vi "Text control 2 v4.8_pump-specific.vi"() -> ()   [LabVIEW 2016]
panel:
  in  "Tab Control":enum32{"Main", "Other parameters"}(tab)
  out "Line running":i32
  out "Total lines":i32
  out "Path":path=path "C:/users/rlp38/09Apr2009LTtesting/test2.txt"
  out "I vs Vg":cluster{"Y data in":dbl[], "X data in":dbl[]}[](graph)
  out "Is":dbl format="%.2e"
  out "Id":dbl format="%.2e"
  out "Ig":dbl format="%.2e"
  out "Id max vs time":cluster{"Y data in":dbl[], "X data in":dbl[]}[](graph)
  out "Id min vs time":cluster{"Y data in":dbl[], "X data in":dbl[]}[](graph)
  out "I vs Vd":cluster{"Y data in":dbl[], "X data in":dbl[]}[](graph)
  in  "Program":string="# Set time units to minutes.\n# Change filenames\n#-------------------------------------------------------\n# Port settings\n# Port 1: Nothing\n# Port 2: To sample\n# Port 3: Ultrapure water\n# Port 4: Nothing\n# Port 5: Nothing\n# Port 6: Nothing\n#-------------------------------------------------------\n# Execution time: 4 x 30 = 120 minutes = 2 hours\n# This script is designed to perform a cycling experiment between two liquids.\n# There are 4 pumping cycles, each one followed by 30 minutes of measurements.\n# All cycles pump ultrapure water (port 3).\n# Flow V = 20 pulses/second (400 ul/min)\n#-------------------------------------------------------\n# Cycle 1\npump /1ZR #initialize pump\npump /1Q #query pump\npump /1? #report absolute plunger position\ntransfer d 1 -1 -0.1 -1 -1 0\nwait-min 1 #wait 1 minute\npump /1N0R #set step resolution: 0.01 mm\npump /1Q #query pump\npump /1? #report absolute plunger position #the plunger should be at 0\nwait 1000 #wait 1 second\npump /1V300R #choose speed: 300 steps/s\npump /1Q #query pump\nwait 1000 #wait 1 second\npump /1O3R #go to port 3, counterclockwise rotation\npump /1Q #query pump\nwait 1000 #wait 1 second\npump /1A2400R #go to absolute position 2400\nwait 20000 #wait 20 seconds\npump /1V20R #set speed to 20 steps/s\npump /1Q #query pump\nwait 10000 # wait 10 seconds\npump /1? #report absolute plunger position #the plunger should have finished moving\npump /1O2R #switch to port 2, counterclockwise rotation\npump /1Q #query pump\nwait 200 #wait 200 milliseconds\npump /1A0R #go to absolute position 0 (= empty syringe)\npump /1Q #query pump\ntransfer d 1 -1 -0.1 -1 -1 0\nwait-min 1\npump /1Q #query pump\npump /1? #report absolute plunger position\ntransfer d 1 -1 -0.1 -1 -1 0\nwait-min 1\npump /1Q #query pump\npump /1? #report absolute plunger position\ntransfer d 1 -1 -0.1 -1 -1 0\nwait-min 1\npump /1Q #query pump\npump /1? #report absolute plunger position\ntransfer d 1 -1 -0.1 -1 -1 0\nwait-min 1\npump /1Q #query pump\npump /1? #report absolute plunger position\ntransfer d 1 -1 -0.1 -1 -1 0\nwait-min 1\npump /1Q #query pump\npump /1? #report absolute plunger position\ntransfer d 1 -1 -0.1 -1 -1 0\nwait-min 1\npump /1Q #query pump\npump /1? #report absolute plunger position\ntransfer d 1 -1 -0.1 -1 -1 0\nwait-min 1\npump /1Q #query pump\npump /1? #report absolute plunger position\ntransfer d 1 -1 -0.1 -1 -1 0\nwait-min 1\npump /1Q #query pump\npump /1? #report absolute plunger position\ntransfer d 1 -1 -0.1 -1 -1 0\nwait-min 1\npump /1Q #query pump\npump /1? #report absolute plunger position\ntransfer d 1 -1 -0.1 -1 -1 0\nwait-min 1\npump /1Q #query pump\npump /1? #report absolute plunger position\ntransfer d 1 -1 -0.1 -1 -1 0\nwait-min 1\npump /1Q #query pump\npump /1? #report absolute plunger position\ntransfer d 1 -1 -0.1 -1 -1 0\nwait-min 1\npump /1Q #query pump\npump /1? #report absolute plunger position\ntransfer d 1 -1 -0.1 -1 -1 0\nwait-min 1\npump /1Q #query pump\npump /1? #report absolute plunger position\ntransfer d 1 -1 -0.1 -1 -1 0\nwait-min 1\npump /1Q #query pump\npump /1? #report absolute plunger position\ntransfer d 1 -1 -0.1 -1 -1 0\nwait-min 1\npump /1Q #query pump\npump /1? #report absolute plunger position\ntransfer d 1 -1 -0.1 -1 -1 0\nwait-min 1\npump /1Q #query pump\npump /1? #report absolute plunger position\ntransfer d 1 -1 -0.1 -1 -1 0\nwait-min 1\npump /1Q #query pump\npump /1? #report absolute plunger position\ntransfer d 1 -1 -0.1 -1 -1 0\nwait-min 1\npump /1Q #query pump\npump /1? #report absolute plunger position\ntransfer d 1 -1 -0.1 -1 -1 0\nwait-min 1\npump /1Q #query pump\npump /1? #report absolute plunger position\ntransfer d 1 -1 -0.1 -1 -1 0\nwait-min 1\npump /1Q #query pump\npump /1? #report absolute plunger position\ntransfer d 1 -1 -0.1 -1 -1 0\nwait-min 1\npump /1Q #query pump\npump /1? #report absolute plunger position\ntransfer d 1 -1 -0.1 -1 -1 0\nwait-min 1\npump /1Q #query pump\npump /1? #report absolute plunger position\ntransfer d 1 -1 -0.1 -1 -1 0\nwait-min 1\npump /1Q #query pump\npump /1? #report absolute plunger position\ntransfer d 1 -1 -0.1 -1 -1 0\nwait-min 1\npump /1Q #query pump\npump /1? #report absolute plunger position\ntransfer d 1 -1 -0.1 -1 -1 0\nwait-min 1\n#-------------------------------------------------------\n# Cycle 2\npump /1ZR #initialize pump\npump /1Q #query pump\npump /1? #report absolute plunger position\ntransfer d 1 -1 -0.1 -1 -1 0\nwait-min 1 #wait 1 minute\npump /1N0R #set step resolution: 0.01 mm\npump /1Q #query pump\npump /1? #report absolute plunger position #the plunger should be at 0\nwait 1000 #wait 1 second\npump /1V300R #choose speed: 300 steps/s\npump /1Q #query pump\nwait 1000 #wait 1 second\npump /1O3R #go to port 3, counterclockwise rotation\npump /1Q #query pump\nwait 1000 #wait 1 second\npump /1A2400R #go to absolute position 2400\nwait 20000 #wait 20 seconds\npump /1V20R #set speed to 20 steps/s\npump /1Q #query pump\nwait 10000 # wait 10 seconds\npump /1? #report absolute plunger position #the plunger should have finished moving\npump /1O2R #switch to port 2, counterclockwise rotation\npump /1Q #query pump\nwait 200 #wait 200 milliseconds\npump /1A0R #go to absolute position 0 (= empty syringe)\npump /1Q #query pump\npump /1? #report absolute plunger position #the plunger should be moving to 0\ntransfer d 1 -1 -0.1 -1 -1 0\nwait-min 1\npump /1Q #query pump\npump /1? #report absolute plunger position\ntransfer d 1 -1 -0.1 -1 -1 0\nwait-min 1\npump /1Q #query pump\npump /1? #report absolute plunger position\ntransfer d 1 -1 -0.1 -1 -1 0\nwait-min 1\npump /1Q #query pump\npump /1? #report absolute plunger position\ntransfer d 1 -1 -0.1 -1 -1 0\nwait-min 1\npump /1Q #query pump\npump /1? #report absolute plunger position\ntransfer d 1 -1 -0.1 -1 -1 0\nwait-min 1\npump /1Q #query pump\npump /1? #report absolute plunger position\ntransfer d 1 -1 -0.1 -1 -1 0\nwait-min 1\npump /1Q #query pump\npump /1? #report absolute plunger position\ntransfer d 1 -1 -0.1 -1 -1 0\nwait-min 1\npump /1Q #query pump\npump /1? #report absolute plunger position\ntransfer d 1 -1 -0.1 -1 -1 0\nwait-min 1\npump /1Q #query pump\npump /1? #report absolute plunger position\ntransfer d 1 -1 -0.1 -1 -1 0\nwait-min 1\npump /1Q #query pump\npump /1? #report absolute plunger position\ntransfer d 1 -1 -0.1 -1 -1 0\nwait-min 1\npump /1Q #query pump\npump /1? #report absolute plunger position\ntransfer d 1 -1 -0.1 -1 -1 0\nwait-min 1\npump /1Q #query pump\npump /1? #report absolute plunger position\ntransfer d 1 -1 -0.1 -1 -1 0\nwait-min 1\npump /1Q #query pump\npump /1? #report absolute plunger position\ntransfer d 1 -1 -0.1 -1 -1 0\nwait-min 1\npump /1Q #query pump\npump /1? #report absolute plunger position\ntransfer d 1 -1 -0.1 -1 -1 0\nwait-min 1\npump /1Q #query pump\npump /1? #report absolute plunger position\ntransfer d 1 -1 -0.1 -1 -1 0\nwait-min 1\npump /1Q #query pump\npump /1? #report absolute plunger position\ntransfer d 1 -1 -0.1 -1 -1 0\nwait-min 1\npump /1Q #query pump\npump /1? #report absolute plunger position\ntransfer d 1 -1 -0.1 -1 -1 0\nwait-min 1\npump /1Q #query pump\npump /1? #report absolute plunger position\ntransfer d 1 -1 -0.1 -1 -1 0\nwait-min 1\npump /1Q #query pump\npump /1? #report absolute plunger position\ntransfer d 1 -1 -0.1 -1 -1 0\nwait-min 1\npump /1Q #query pump\npump /1? #report absolute plunger position\ntransfer d 1 -1 -0.1 -1 -1 0\nwait-min 1\npump /1Q #query pump\npump /1? #report absolute plunger position\ntransfer d 1 -1 -0.1 -1 -1 0\nwait-min 1\npump /1Q #query pump\npump /1? #report absolute plunger position\ntransfer d 1 -1 -0.1 -1 -1 0\nwait-min 1\npump /1Q #query pump\npump /1? #report absolute plunger position\ntransfer d 1 -1 -0.1 -1 -1 0\nwait-min 1\npump /1Q #query pump\npump /1? #report absolute plunger position\ntransfer d 1 -1 -0.1 -1 -1 0\nwait-min 1\npump /1Q #query pump\npump /1? #report absolute plunger position\ntransfer d 1 -1 -0.1 -1 -1 0\nwait-min 1\n#-------------------------------------------------------\n# Cycle 3\npump /1ZR #initialize pump\npump /1Q #query pump\npump /1? #report absolute plunger position\ntransfer d 1 -1 -0.1 -1 -1 0\nwait-min 1 #wait 1 minute\npump /1N0R #set step resolution: 0.01 mm\npump /1Q #query pump\npump /1? #report absolute plunger position #the plunger should be at 0\nwait 1000 #wait 1 second\npump /1V300R #choose speed: 300 steps/s\npump /1Q #query pump\nwait 1000 #wait 1 second\npump /1O3R #go to port 3, counterclockwise rotation\npump /1Q #query pump\nwait 1000 #wait 1 second\npump /1A2400R #go to absolute position 2400\nwait 20000 #wait 20 seconds\npump /1V20R #set speed to 20 steps/s\npump /1Q #query pump\nwait 10000 # wait 10 seconds\npump /1? #report absolute plunger position #the plunger should have finished moving\npump /1O2R #switch to port 2, counterclockwise rotation\npump /1Q #query pump\nwait 200 #wait 200 milliseconds\npump /1A0R #go to absolute position 0 (= empty syringe)\npump /1Q #query pump\npump /1? #report absolute plunger position #the plunger should be moving to 0\ntransfer d 1 -1 -0.1 -1 -1 0\nwait-min 1\npump /1Q #query pump\npump /1? #report absolute plunger position\ntransfer d 1 -1 -0.1 -1 -1 0\nwait-min 1\npump /1Q #query pump\npump /1? #report absolute plunger position\ntransfer d 1 -1 -0.1 -1 -1 0\nwait-min 1\npump /1Q #query pump\npump /1? #report absolute plunger position\ntransfer d 1 -1 -0.1 -1 -1 0\nwait-min 1\npump /1Q #query pump\npump /1? #report absolute plunger position\ntransfer d 1 -1 -0.1 -1 -1 0\nwait-min 1\npump /1Q #query pump\npump /1? #report absolute plunger position\ntransfer d 1 -1 -0.1 -1 -1 0\nwait-min 1\npump /1Q #query pump\npump /1? #report absolute plunger position\ntransfer d 1 -1 -0.1 -1 -1 0\nwait-min 1\npump /1Q #query pump\npump /1? #report absolute plunger position\ntransfer d 1 -1 -0.1 -1 -1 0\nwait-min 1\npump /1Q #query pump\npump /1? #report absolute plunger position\ntransfer d 1 -1 -0.1 -1 -1 0\nwait-min 1\npump /1Q #query pump\npump /1? #report absolute plunger position\ntransfer d 1 -1 -0.1 -1 -1 0\nwait-min 1\npump /1Q #query pump\npump /1? #report absolute plunger position\ntransfer d 1 -1 -0.1 -1 -1 0\nwait-min 1\npump /1Q #query pump\npump /1? #report absolute plunger position\ntransfer d 1 -1 -0.1 -1 -1 0\nwait-min 1\npump /1Q #query pump\npump /1? #report absolute plunger position\ntransfer d 1 -1 -0.1 -1 -1 0\nwait-min 1\npump /1Q #query pump\npump /1? #report absolute plunger position\ntransfer d 1 -1 -0.1 -1 -1 0\nwait-min 1\npump /1Q #query pump\npump /1? #report absolute plunger position\ntransfer d 1 -1 -0.1 -1 -1 0\nwait-min 1\npump /1Q #query pump\npump /1? #report absolute plunger position\ntransfer d 1 -1 -0.1 -1 -1 0\nwait-min 1\npump /1Q #query pump\npump /1? #report absolute plunger position\ntransfer d 1 -1 -0.1 -1 -1 0\nwait-min 1\npump /1Q #query pump\npump /1? #report absolute plunger position\ntransfer d 1 -1 -0.1 -1 -1 0\nwait-min 1\npump /1Q #query pump\npump /1? #report absolute plunger position\ntransfer d 1 -1 -0.1 -1 -1 0\nwait-min 1\npump /1Q #query pump\npump /1? #report absolute plunger position\ntransfer d 1 -1 -0.1 -1 -1 0\nwait-min 1\npump /1Q #query pump\npump /1? #report absolute plunger position\ntransfer d 1 -1 -0.1 -1 -1 0\nwait-min 1\npump /1Q #query pump\npump /1? #report absolute plunger position\ntransfer d 1 -1 -0.1 -1 -1 0\nwait-min 1\npump /1Q #query pump\npump /1? #report absolute plunger position\ntransfer d 1 -1 -0.1 -1 -1 0\nwait-min 1\npump /1Q #query pump\npump /1? #report absolute plunger position\ntransfer d 1 -1 -0.1 -1 -1 0\nwait-min 1\npump /1Q #query pump\npump /1? #report absolute plunger position\ntransfer d 1 -1 -0.1 -1 -1 0\nwait-min 1\n#-------------------------------------------------------\n# Cycle 4\npump /1ZR #initialize pump\npump /1Q #query pump\npump /1? #report absolute plunger position\ntransfer d 1 -1 -0.1 -1 -1 0\nwait-min 1 #wait 1 minute\npump /1N0R #set step resolution: 0.01 mm\npump /1Q #query pump\npump /1? #report absolute plunger position #the plunger should be at 0\nwait 1000 #wait 1 second\npump /1V300R #choose speed: 300 steps/s\npump /1Q #query pump\nwait 1000 #wait 1 second\npump /1O3R #go to port 3, counterclockwise rotation\npump /1Q #query pump\nwait 1000 #wait 1 second\npump /1A2400R #go to absolute position 2400\nwait 20000 #wait 20 seconds\npump /1V20R #set speed to 20 steps/s\npump /1Q #query pump\nwait 10000 # wait 10 seconds\npump /1? #report absolute plunger position #the plunger should have finished moving\npump /1O2R #switch to port 2, counterclockwise rotation\npump /1Q #query pump\nwait 200 #wait 200 milliseconds\npump /1A0R #go to absolute position 0 (= empty syringe)\npump /1Q #query pump\npump /1? #report absolute plunger position #the plunger should be moving to 0\ntransfer d 1 -1 -0.1 -1 -1 0\nwait-min 1\npump /1Q #query pump\npump /1? #report absolute plunger position\ntransfer d 1 -1 -0.1 -1 -1 0\nwait-min 1\npump /1Q #query pump\npump /1? #report absolute plunger position\ntransfer d 1 -1 -0.1 -1 -1 0\nwait-min 1\npump /1Q #query pump\npump /1? #report absolute plunger position\ntransfer d 1 -1 -0.1 -1 -1 0\nwait-min 1\npump /1Q #query pump\npump /1? #report absolute plunger position\ntransfer d 1 -1 -0.1 -1 -1 0\nwait-min 1\npump /1Q #query pump\npump /1? #report absolute plunger position\ntransfer d 1 -1 -0.1 -1 -1 0\nwait-min 1\npump /1Q #query pump\npump /1? #report absolute plunger position\ntransfer d 1 -1 -0.1 -1 -1 0\nwait-min 1\npump /1Q #query pump\npump /1? #report absolute plunger position\ntransfer d 1 -1 -0.1 -1 -1 0\nwait-min 1\npump /1Q #query pump\npump /1? #report absolute plunger position\ntransfer d 1 -1 -0.1 -1 -1 0\nwait-min 1\npump /1Q #query pump\npump /1? #report absolute plunger position\ntransfer d 1 -1 -0.1 -1 -1 0\nwait-min 1\npump /1Q #query pump\npump /1? #report absolute plunger position\ntransfer d 1 -1 -0.1 -1 -1 0\nwait-min 1\npump /1Q #query pump\npump /1? #report absolute plunger position\ntransfer d 1 -1 -0.1 -1 -1 0\nwait-min 1\npump /1Q #query pump\npump /1? #report absolute plunger position\ntransfer d 1 -1 -0.1 -1 -1 0\nwait-min 1\npump /1Q #query pump\npump /1? #report absolute plunger position\ntransfer d 1 -1 -0.1 -1 -1 0\nwait-min 1\npump /1Q #query pump\npump /1? #report absolute plunger position\ntransfer d 1 -1 -0.1 -1 -1 0\nwait-min 1\npump /1Q #query pump\npump /1? #report absolute plunger position\ntransfer d 1 -1 -0.1 -1 -1 0\nwait-min 1\npump /1Q #query pump\npump /1? #report absolute plunger position\ntransfer d 1 -1 -0.1 -1 -1 0\nwait-min 1\npump /1Q #query pump\npump /1? #report absolute plunger position\ntransfer d 1 -1 -0.1 -1 -1 0\nwait-min 1\npump /1Q #query pump\npump /1? #report absolute plunger position\ntransfer d 1 -1 -0.1 -1 -1 0\nwait-min 1\npump /1Q #query pump\npump /1? #report absolute plunger position\ntransfer d 1 -1 -0.1 -1 -1 0\nwait-min 1\npump /1Q #query pump\npump /1? #report absolute plunger position\ntransfer d 1 -1 -0.1 -1 -1 0\nwait-min 1\npump /1Q #query pump\npump /1? #report absolute plunger position\ntransfer d 1 -1 -0.1 -1 -1 0\nwait-min 1\npump /1Q #query pump\npump /1? #report absolute plunger position\ntransfer d 1 -1 -0.1 -1 -1 0\nwait-min 1\npump /1Q #query pump\npump /1? #report absolute plunger position\ntransfer d 1 -1 -0.1 -1 -1 0\nwait-min 1\npump /1Q #query pump\npump /1? #report absolute plunger position\ntransfer d 1 -1 -0.1 -1 -1 0\nwait-min 1\n#-------------------------------------------------------"
  out "Command running:":string="#output s 0 0 0 -0.008 0.008 0.002"
  out "Serial port data":string
  out "Elapsed Time":dbl caption="Elapsed Time (s)"
  in  "Units":u16(ring)=1 items=["Seconds", "Minutes", "Hours"]
  in  "Time Offset":dbl caption="Set Start Time (s)"
  in  "Reset":bool
  in  "Auto Reset":bool
  in  "integration time":u32(slide) max=2 step=1 scale=0.0..2.0
  in  "Interrupt run":bool
  out "Absolute plunger position vs time":cluster{"Y data in":dbl[], "X data in":dbl[]}[](graph)
  out "Valve position vs time":cluster{"Y data in":dbl[], "X data in":dbl[]}[](graph)
  in  "Halt pump":bool
  in  "Hard stop pump":bool
  in  "Gate Range\nmode":u16(ring) items=["Auto", "Limited", "Fixed"]
  in  "Gate Range":u8(slide)=6 max=11 scale=0.0..11.0
  in  "Source/Drain\nRange mode":u16(ring) items=["Auto", "Limited", "Fixed"]
  in  "Source/Drain Range":u8(slide)=6 max=11 scale=0.0..11.0
  in  "Panel Controls":T1={"Emergency Stop"=refnum, "TransGraph Max"=1e-05, "Text/Graph (text=false)"=TRUE} {"TransGraph Max" format="%.2e"}
  in  "Panel Controls 2":T2={"Emergency Stop"=refnum, "TransGraph Max"=1e-05, "Text/Graph (text=false)"=TRUE, "TransGraph Min"=1e-11} {"TransGraph Min" format="%.2e"; "TransGraph Max" format="%.2e"}
  in  "SMU4":cluster{"on/off":bool, "Voltage":dbl} {"Voltage" min=-100.0 max=100.0 format="%.2f"}
  in  "Full Reset":bool
  in  "Standby":T3
  out "error out":errorcluster
  in  "Delay before read (ms)":u32=1000
  in  "byte count":u32=64
  in  "Serial End Mode for Reads":u16(ring)=2 items=["None", "LastBit", "TermChar"]
  in  "Timeout (ms)":u32=10000
  in  "Enable Termination\nChar (T)":bool=TRUE
  in  "Termination char\n(0xA = '\\n' = LF)\n(0xD = '\\r' = CR)":u8=13 format="%.0x"
  in  "flow control":u16(ring) items=["None"=0, "XON/XOFF"=1, "RTS/CTS"=2, "DTR/DSR"=4]
  in  "stop bits":u16(ring)=10 items=["1.0"=10, "1.5"=15, "2.0"=20]
  in  "parity":u16(ring) items=["None", "Odd", "Even", "Mark", "Space"]
  in  "data bits":u16=8 min=5 max=8 step=1
  in  "VISA resource name":refnum<visa-resource-name>="COM6"
  in  "baud rate":u32=9600
  in  "Drain: Compliance":dbl=0.001 format="%.8f"
  in  "Gate: Compliance":dbl=0.001 format="%.8f"
  in  "hold time /s":dbl format="%.2f"
  in  "delay time /s":dbl format="%.2f"
  in  "Integration time (short)":dbl=0.0019 min=8e-05 max=0.0019 step=8e-05 format="%^.0e"
  in  "Integration time (long)":dbl=0.32 min=0.04 max=2.0 step=0.02 format="%.2f"
  in  "Step delay /s":dbl format="%.2f"
  in  "Prefix (transfer)":string="_step_1_ultrapure_H2O_"
  in  "Suffix (transfer)":string="_T.txt"
  in  "Prefix (Idmax-Idmin)":string="_step_1_ultrapure_H2O_Idmax_Idmin_vs_time_Vg=-1.0V_Vd=-1.0V"
  in  "Suffix (Idmax-Idmin)":string=".txt"
  in  "Prefix (output)":string="_step_1_ultrapure_H2O_"
  in  "Suffix (output)":string="_O.txt"
  in  "Prefix (script)":string="_step_1_ultrapure_H2O_script"
  in  "Prefix (serial port output)":string="_step_1_ultrapure_H2O_serial port output"
  in  "Prefix (plunger)":string="_step_1_ultrapure_H2O_plunger_vs_time"
  in  "Suffix (plunger)":string=".txt"
  in  "Gate":T4={"Gate Start"=0.0, "Gate Stop"=2.0, "Gate Step (linear only)"=1.0, "Gate Compliance"=0.0001, "Gate PComp"=0.0, "Range mode"=0, "Range"=6} {"Range" max=11 scale=0.0..11.0; "Range mode" items=["Auto", "Limited", "Fixed"]; "Gate PComp" format="%^.2e"; "Gate Compliance" format="%^.2e"; "Gate Step (linear only)" format="%^.4e"; "Gate Stop" format="%^.4e"; "Gate Start" format="%^.4e"}
  in  "Drain 2":T5={"Drain Start"=0.0, "Drain Stop"=2.0, "Drain Compliance"=0.0001, "Drain Step"=1.0, "Drain PComp"=0.0, "Range mode"=0, "Range"=6} {"Range" max=11 scale=0.0..11.0; "Range mode" items=["Auto", "Limited", "Fixed"]; "Drain PComp" format="%^.2e"; "Drain Step" format="%^.4e"; "Drain Compliance" format="%^.2e"; "Drain Stop" format="%^.4e"; "Drain Start" format="%^.4e"}
  in  "Timings 2":T6={"integration time"=0, "Short/Long integration time"=0.00064, "hold time (sec)"=0.0, "delay time (sec)"=0.0, "Step Time (0 disables)"=0.0, "sweep method"=0, "Pulse period"=0.005, "Base voltage"=0.0, "Pulse width"=0.0005} {"Pulse width" min=0.0005 max=0.1 step=0.0001 format="%.4f"; "Base voltage" format="%^.4e"; "Pulse period" min=0.005 max=1.0 step=0.0001 format="%.4f"; "sweep method" items=["Continuous", "Pulsed"]; "Step Time (0 disables)" format="%.2f"; "delay time (sec)" format="%.4f"; "hold time (sec)" format="%.4f"; "Short/Long integration time" format="%^.0e"; "integration time" scale=0.0..2.0}
  # "Syntax:\nitime [s|m|l]\ngaterangemode [a|l|f]\ndrainrangemode [a|l|f]\npulsed [on|off] PulsePeriod(sec) PulseBaseVoltage PulseONWidth(sec)\nstandby [on l off]\nwait NumMilliseconds\nwait-min NumMinutes\n# texthere = comment\ntransfer [s|d] VgStart VgStop VgStep VdStart VdStop VdStep\noutput [s|d] VgStart VgStop VgStep VdStart VdStop VdStep\nsample Vg Vd NumSamples Time(s) SampleInterval(s)\nsamplei Idg NumSamples Time(s) SampleInterval(s) VDGcompliance\n100 samples is approximately 13 seconds with medium integration\n# if in doubt use SampleInterval(s) = 0.004\nstressV VG VD IGcompliance IDcompliance Duration(sec)\nstressI IDG VDGcompliance Duration(sec)\nvsu2pulse Bias Duration(s)\npulsedstressV [s|d] VEstop VgON VgOFF Period(s) PulseONwidth(s) Vd\nsample-fpp Vg Vd NumSamples Time\nresample-fpp Vg Vd\ntransfer-fpp [s|d] VgStart VgStop VgStep VdStart VdStop VdStep\noutput-fpp [s|d] VgStart VgStop VgStep VdStart VdStop VdStep\nserial SerialPortCommand\npump SerialPortCommand for the OEM pump\n\nSPM OEM Pump Syntax (<x>: pump number, use 1 if only one pump):\nif the command syntax contains [R], then append the letter R to the command\n/<x>Q: query (a query command should follow each command)\n/<x>Z[R] or /<x>Y[R]: initialize pump\n/<x>N<n>[R] (<n>=0,1): <0> (<1>) microstep 0.01 mm (0.00125 mm) resolution\n/<x>I<n> (<n>=0-6): turn to port number n (clockwise)\n/<x>O<n> (<n>=0-6): turn to port number n (counterclockwise)\n/<x>X: Re-execute last command string\n/<x>G<n>[R] (<n>=0-60000): repeat command sequence (default: 0, 0=loop forever)\n/<x>g: Mark the start of a repeat sequence (max = 10)\n/<x>M<n>[R] (<n>=0-86400000): delay command execution by n milliseconds\n/<x>H: Halt; Pause the sequence after finishing the current move\n/<x>T: Hardstop; Interrupt the current move and suppress it from the sequence\n/<x>A<n>[R] (<n>=0-3000 with N=0, 0-24000 with N=1): absolute position\n/<x>P<n>[R] (<n>=0-3000 with N=0, 0-24000 with N=1): relative pickup\n/<x>D<n>[R] (<n>=0-3000 with N=0, 0-24000 with N=1): relative dispense\n/<x>V<n>[R] (<n>=5-1600 default: 150): set peak speed (pulses/sec)\n/<x>S<n>[R] (<n>=10-40 default: 22): set speed (NOT in pulses/sec, look in manual)\nNOTE: When controlled with absolute position, one does not need to pay special attention to the syringe that is mounted on the pump.\nWithdraw from lower stage (ports 3, 5), dispense from higher stage (ports 2, 4, 6).\nConnect Port 1 to waste."
  # "Time"
  # "1\n2\n3\n4\n5\n6\n7\n8\n9\n10\n11\n12\n13\n14\n15\n16\n17\n18\n19\n20"
  # "Serial port settings"
  # "Filename settings"
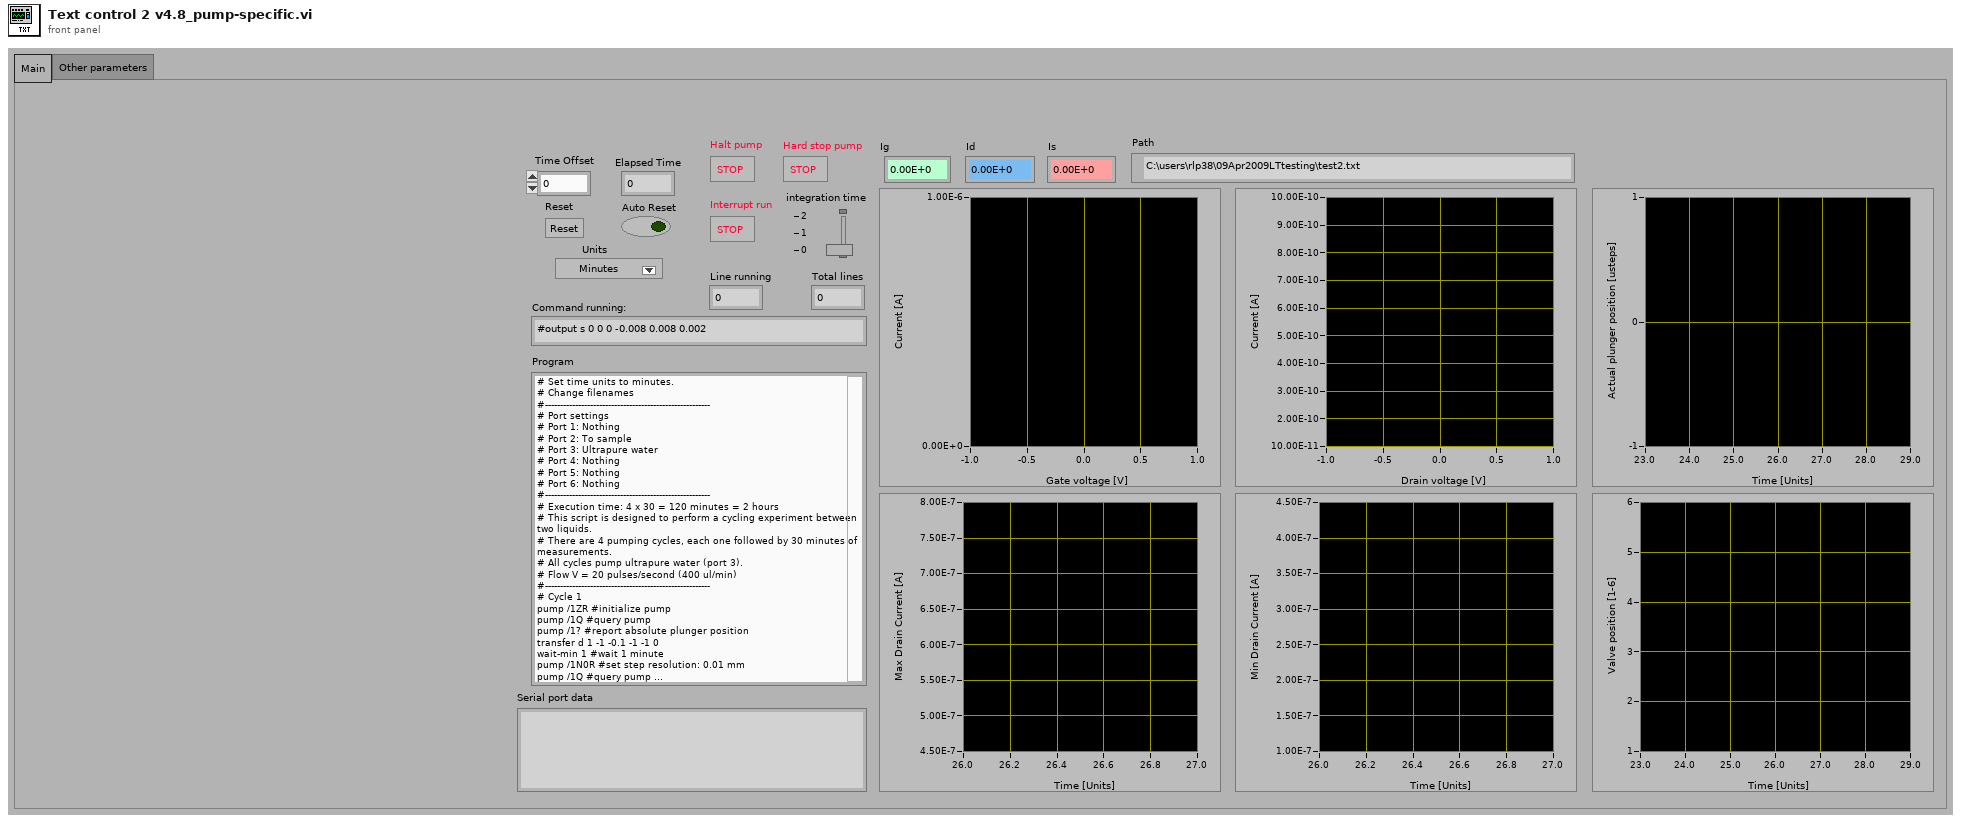
[diagram p1: front panel]
types:
  T1 = cluster{"Emergency Stop":refnum<vi>, "TransGraph Max":dbl, "Text/Graph (text=false)":bool}
  T2 = cluster{"Emergency Stop":refnum<vi>, "TransGraph Max":dbl, "Text/Graph (text=false)":bool, "TransGraph Min":dbl}
  T3 = cluster{"Gate Standby":bool, "Drain Standby":bool}
  T4 = cluster{"Gate Start":dbl, "Gate Stop":dbl, "Gate Step (linear only)":dbl, "Gate Compliance":dbl, "Gate PComp":dbl, "Range mode":u16, "Range":u8}
  T5 = cluster{"Drain Start":dbl, "Drain Stop":dbl, "Drain Compliance":dbl, "Drain Step":dbl, "Drain PComp":dbl, "Range mode":u16, "Range":u8}
  T6 = cluster{"integration time":u32, "Short/Long integration time":dbl, "hold time (sec)":dbl, "delay time (sec)":dbl, "Step Time (0 disables)":dbl, "sweep method":u16, "Pulse period":dbl, "Base voltage":dbl, "Pulse width":dbl}
  T7 = enum16{"open", "replace", "create", "open or create", "replace or create", "replace or create with confirmation"}
  T8 = cluster{"V2 Start":dbl, "V2 Step":dbl, "Number of points":i32}
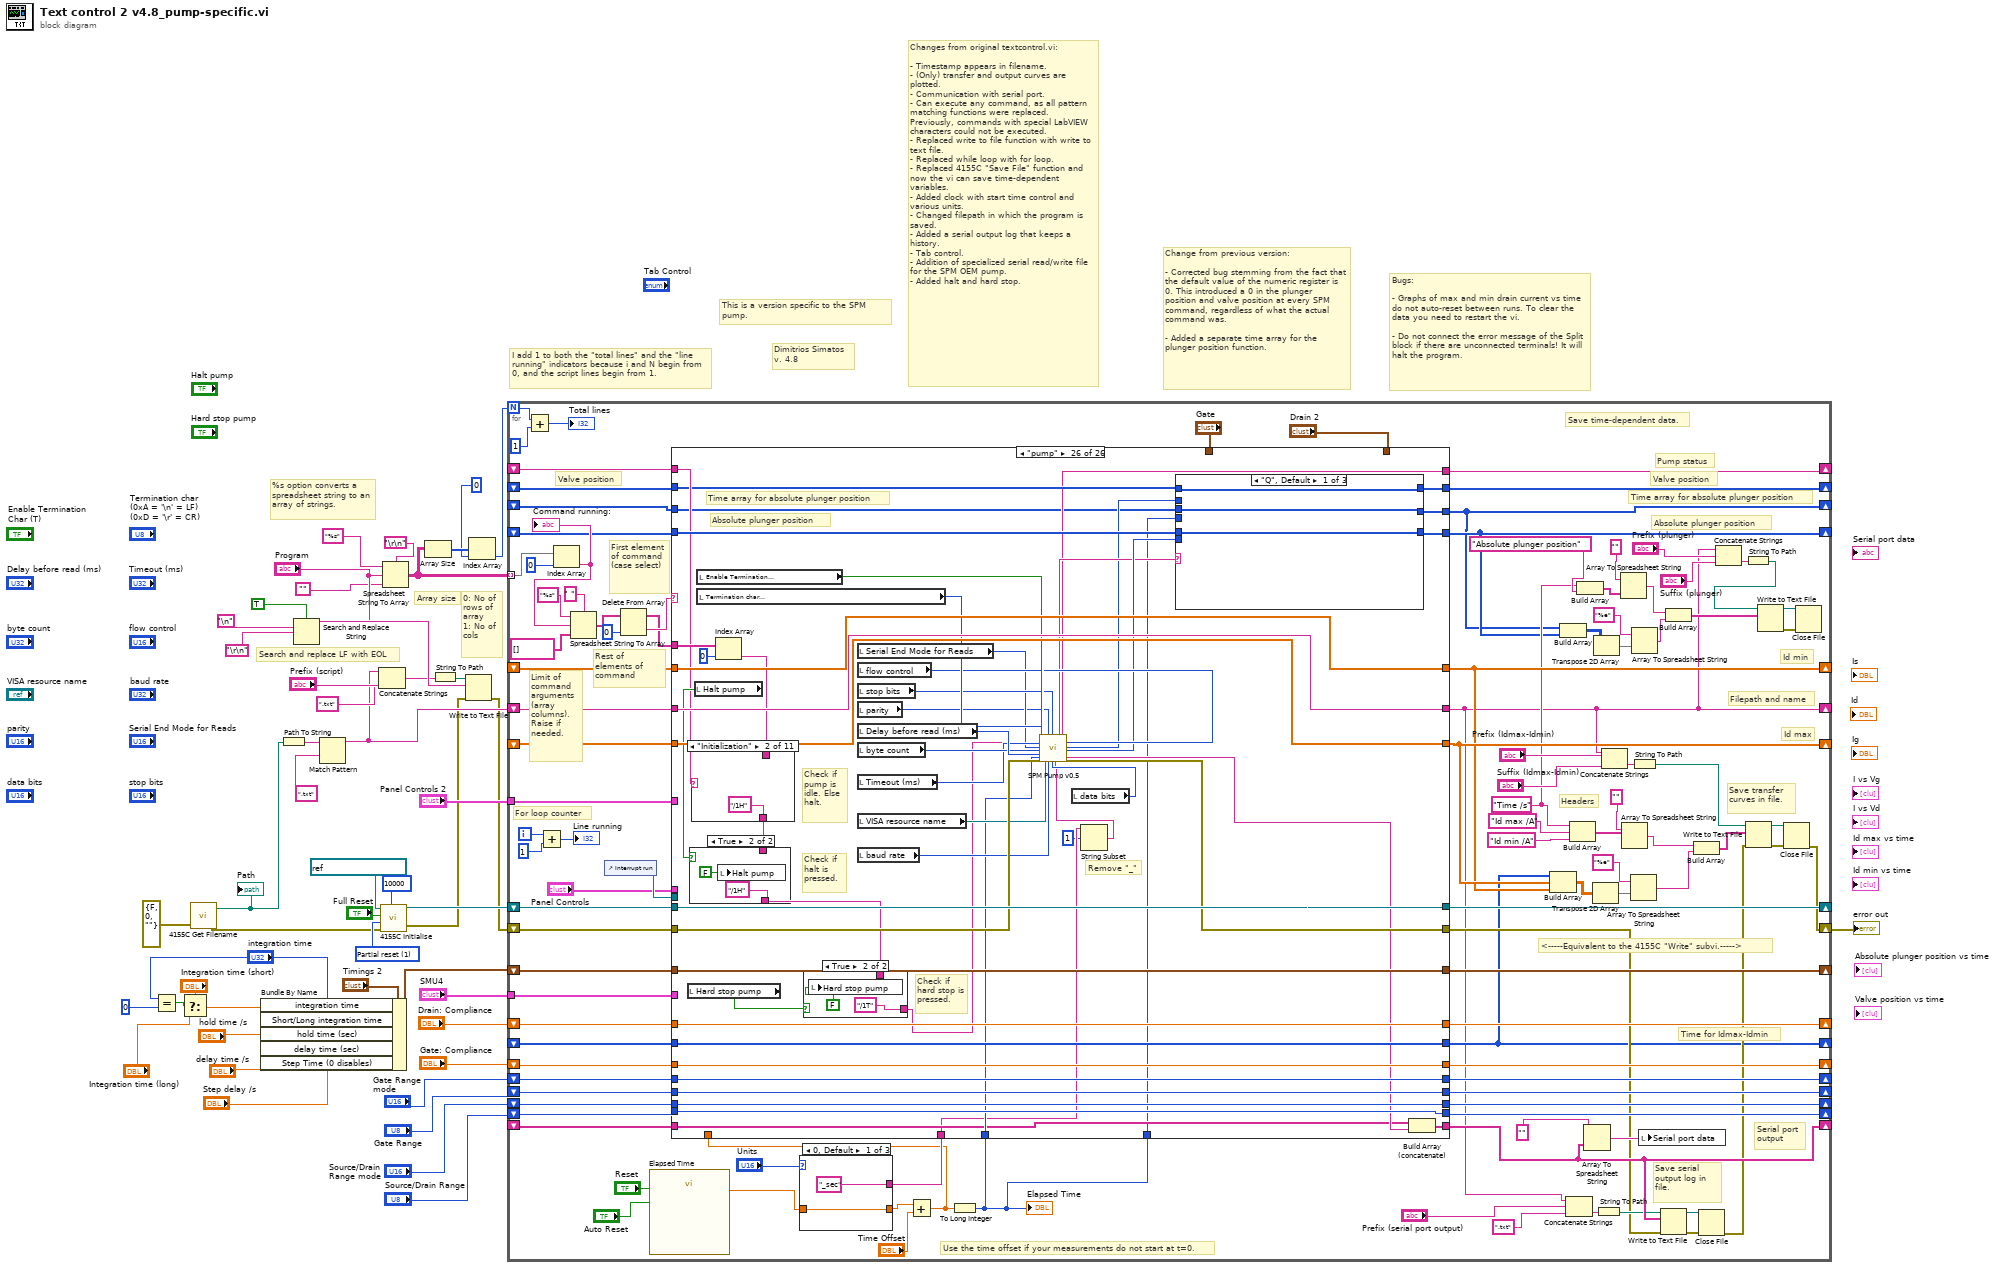
[diagram p0: block diagram]
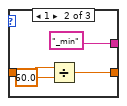
[diagram p2: hidden frame]
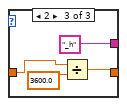
[diagram p3: hidden frame]
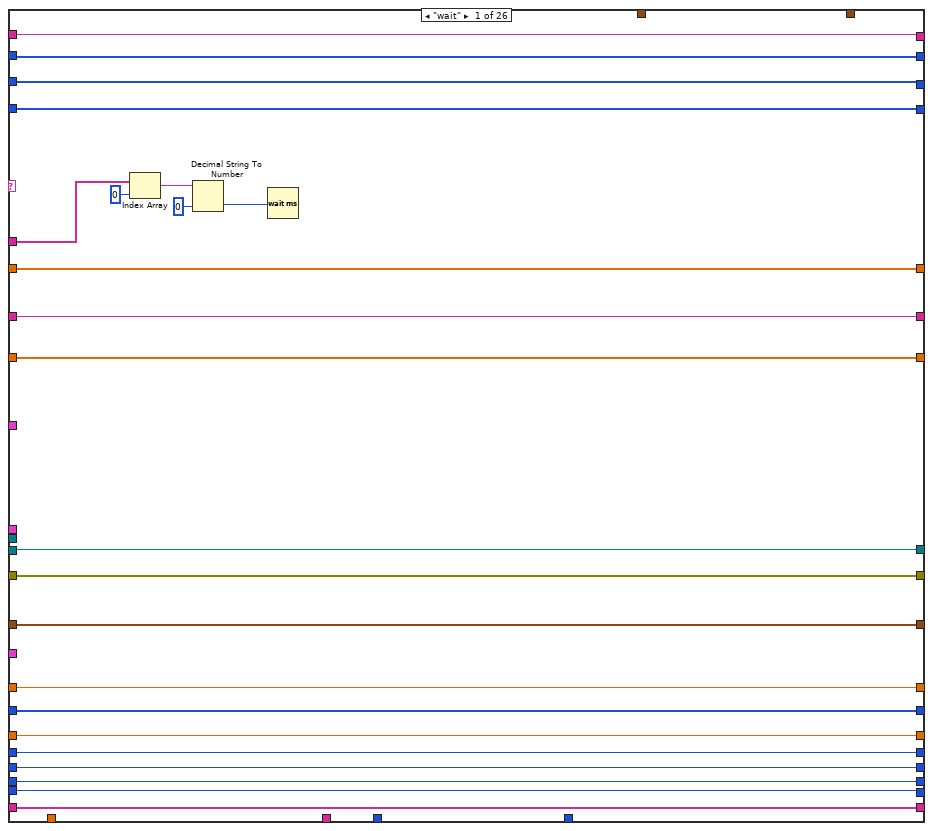
[diagram p4: hidden frame]
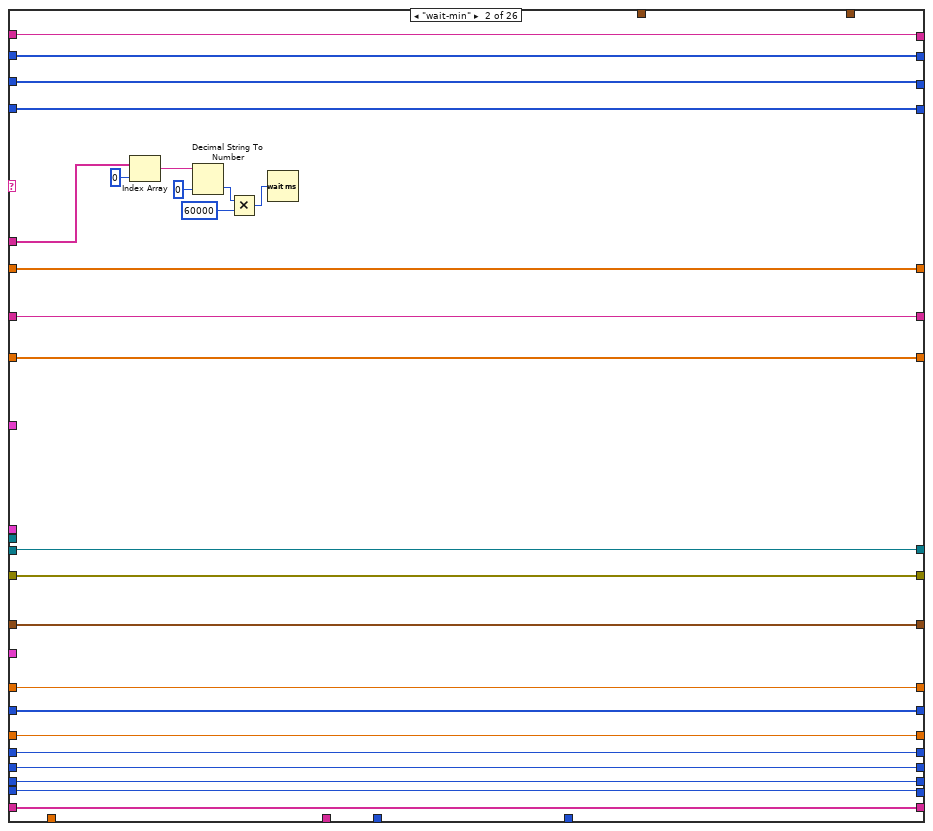
[diagram p5: hidden frame]
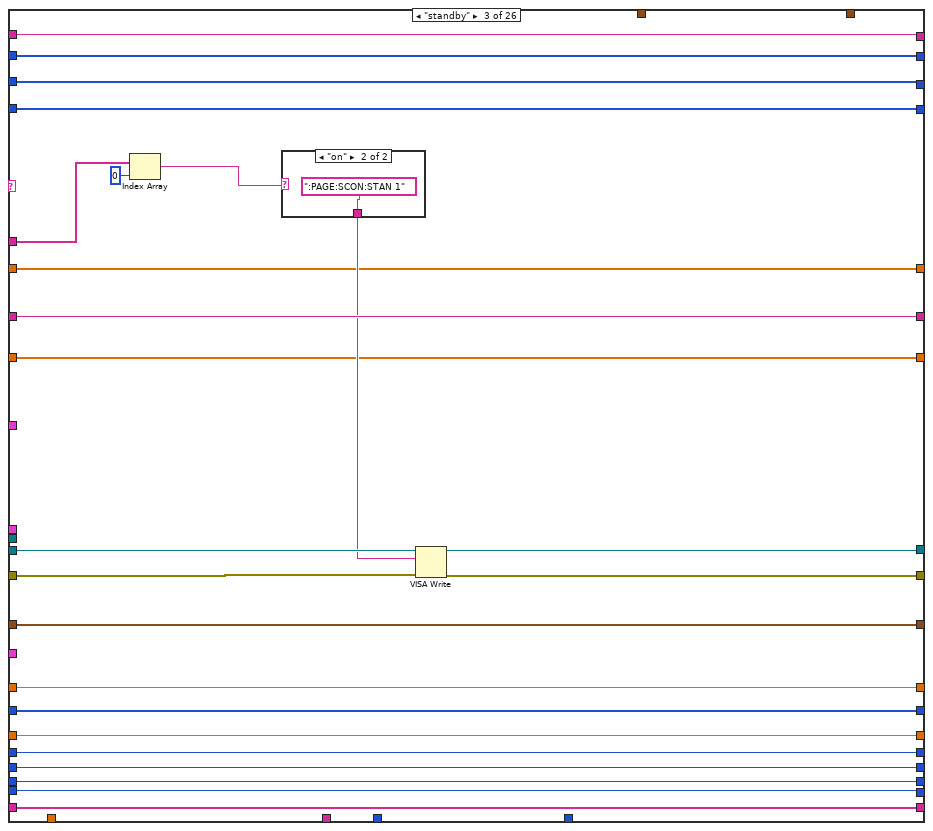
[diagram p6: hidden frame]
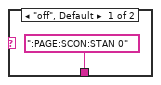
[diagram p7: hidden frame]
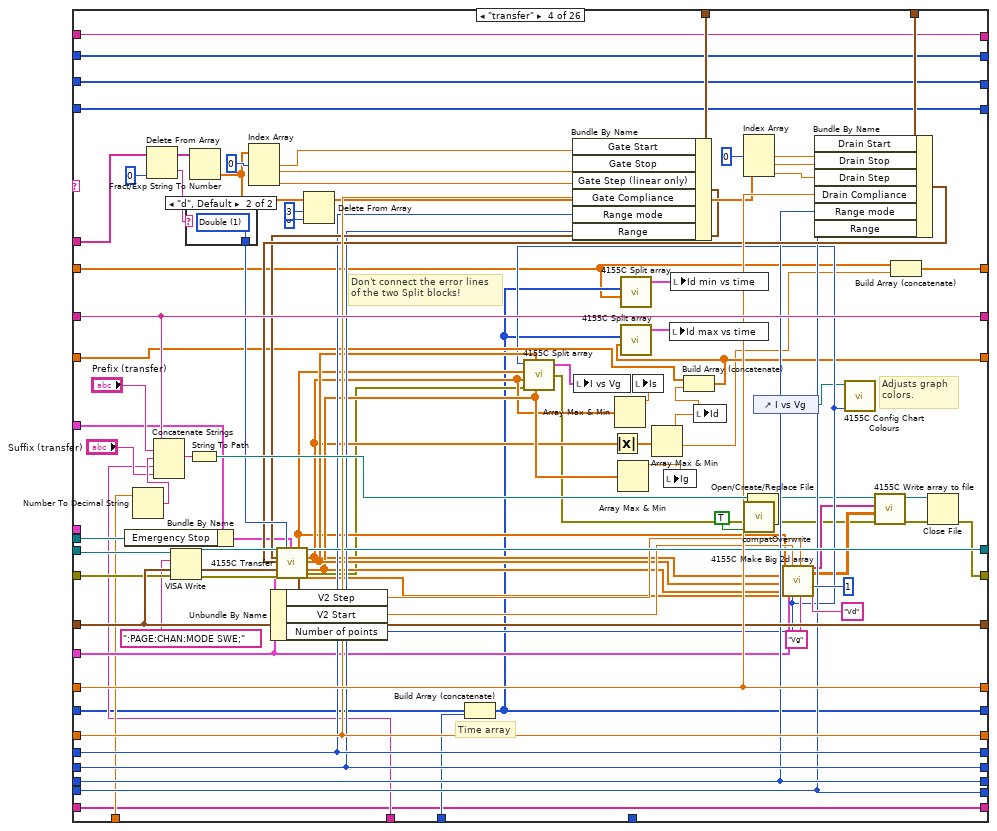
[diagram p8: hidden frame]
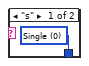
[diagram p9: hidden frame]
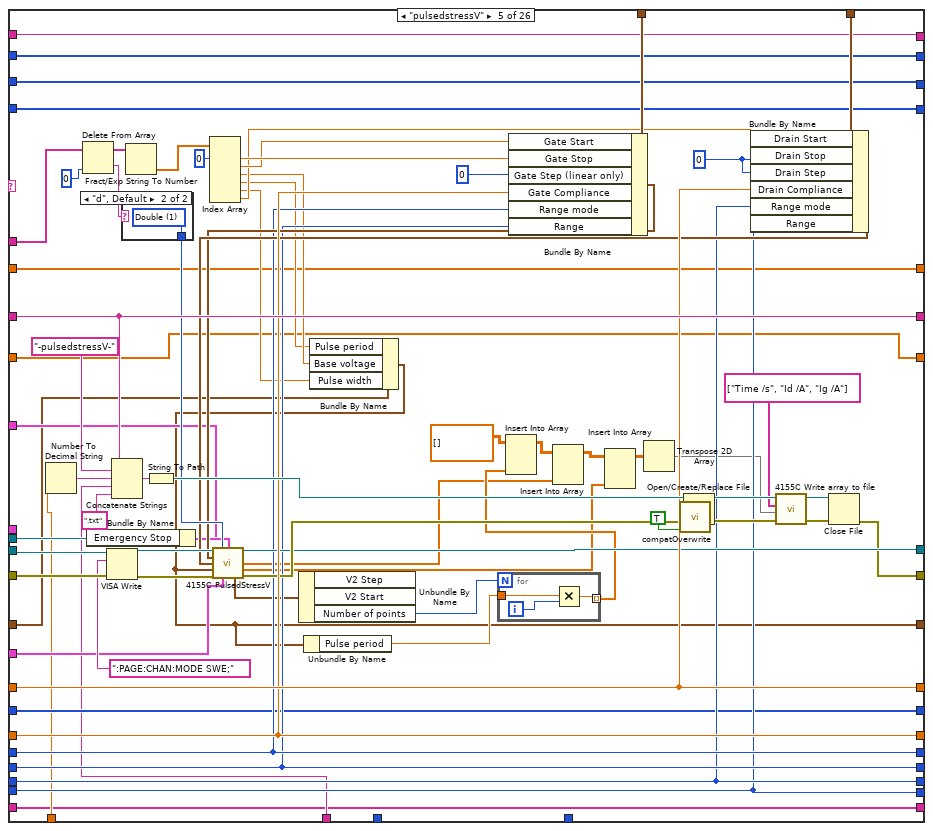
[diagram p10: hidden frame]
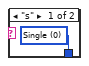
[diagram p11: hidden frame]
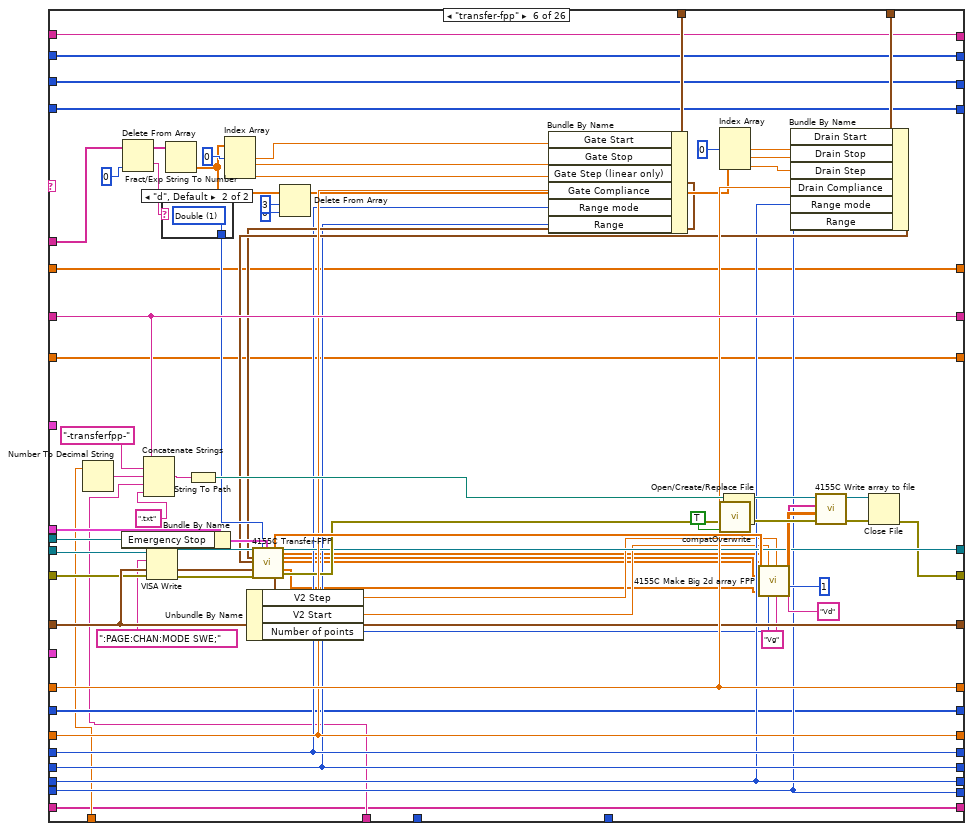
[diagram p12: hidden frame]
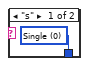
[diagram p13: hidden frame]
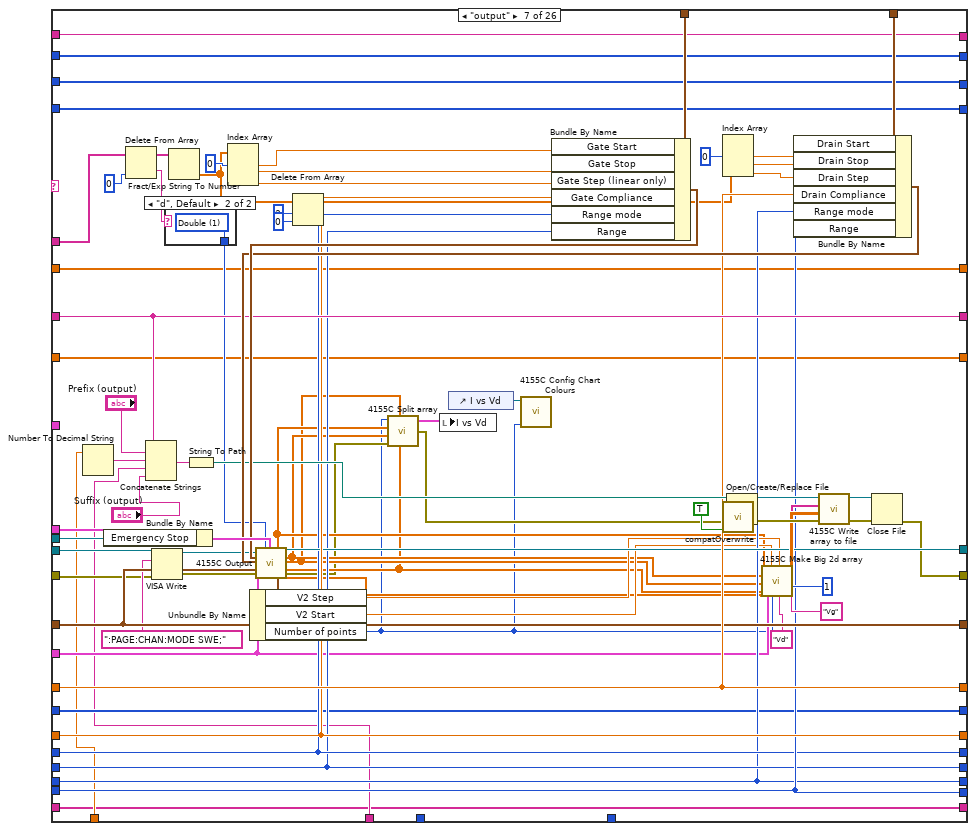
[diagram p14: hidden frame]
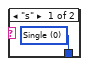
[diagram p15: hidden frame]
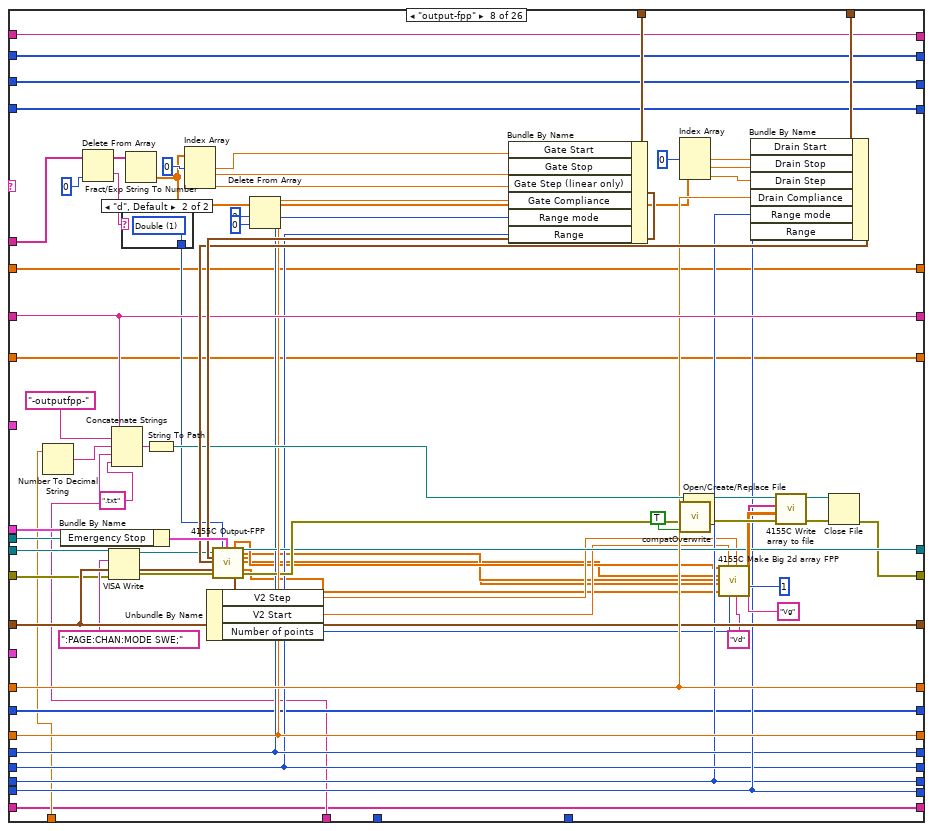
[diagram p16: hidden frame]
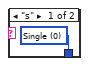
[diagram p17: hidden frame]
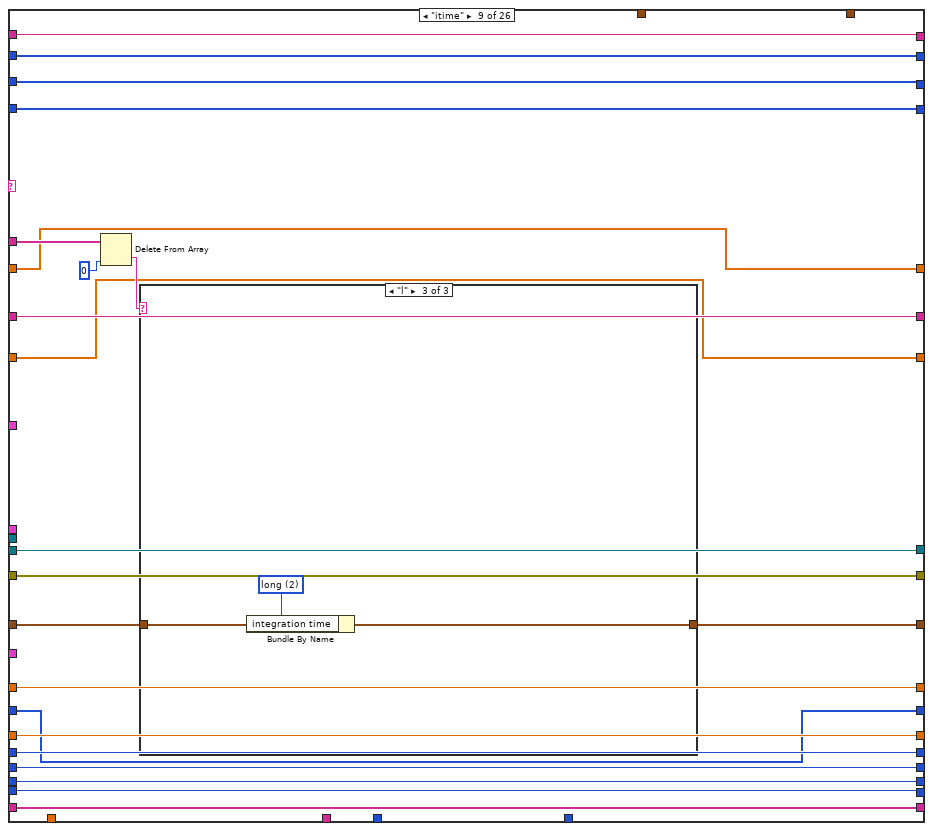
[diagram p18: hidden frame]
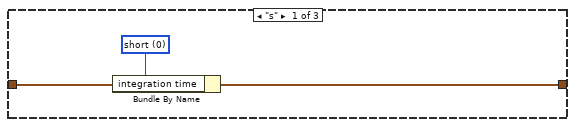
[diagram p19: hidden frame]
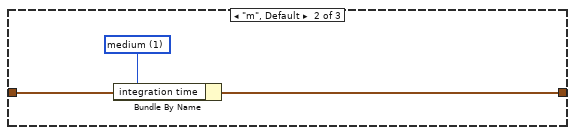
[diagram p20: hidden frame]
diagram:
  w40 = u16 1 items=["Reset All", "Partial reset"] ("Type of reset")
  # "Change from previous version:\n\n- Corrected bug stemming from the fact that the default value of the numeric register is 0. This introduced a 0 in the plunger position and valve position at every SPM command, regardless of what the actual command was.\n\n- Added a separate time array for the plunger position function."
  # "This is a version specific to the SPM pump."
  # "I add 1 to both the \"total lines\" and the \"line running\" indicators because i and N begin from 0, and the script lines begin from 1."
  # "Bugs:\n\n- Graphs of max and min drain current vs time do not auto-reset between runs. To clear the data you need to restart the vi.\n\n- Do not connect the error message of the Split block if there are unconnected terminals! It will halt the program."
  # "Array size"
  # "%s option converts a spreadsheet string to an array of strings."
  # "0: No of rows of array\n1: No of cols"
  # "Dimitrios Simatos\nv. 4.8"
  # "Changes from original textcontrol.vi:\n\n- Timestamp appears in filename.\n- (Only) transfer and output curves are plotted.\n- Communication with serial port.\n- Can execute any command, as all pattern matching functions were replaced. Previously, commands with special LabVIEW characters could not be executed.\n- Replaced write to file function with write to text file.\n- Replaced while loop with for loop.\n- Replaced 4155C \"Save File\" function and now the vi can save time-dependent variables.\n- Added clock with start time control and various units.\n- Changed filepath in which the program is saved.\n- Added a serial output log that keeps a history.\n- Tab control.\n- Addition of specialized serial read/write file for the SPM OEM pump.\n- Added halt and hard stop."
  # "Search and replace LF with EOL"
  n1 = Equal?(x="integration time", y=u32 0) -> (x = y?=w44:bool)
  n2 = Select(t="Integration time (short)", s=w44, f="Integration time (long)") -> (s? t:f=w48:dbl)
  n3 = call "4155C Get Filename.vi"("error in (no error)"=errorcluster {"status"=FALSE, "code"=0, "source"=""}) -> ("error out"=w35:errorcluster, "path"=w10:path)  [unwired: 2 in, 1 out]
  "Path" <- w10
  n4 = Bundle By Name(cluster="Timings 2", "integration time"="integration time", "Short/Long integration time"=w48, "hold time (sec)"="hold time /s", "delay time (sec)"="delay time /s", "Step Time (0 disables)"="Step delay /s") -> (w33:T6)
  n5 = Path To String(path=w10) -> (string=w11:string)
  n6 = Search and Replace String(replace all?=TRUE ("replace all? (F)"), input string="Program", search string="\n", replace string="\r\n") -> (result string=w23:string)  [unwired: 4 in, 3 out]
  n7 = Match Pattern(string=w11, regular expression=".txt") -> (before substring=w5:string)  [unwired: 1 in, 3 out]
  n8 = Concatenate Strings(w5, "Prefix (script)", ".txt" ("regular expression")) -> (w4:string)
  n9 = call "4155C Initialise.vi"("VISA resource name in"=refnum<visa-resource-name> "GPIB0::14::INSTR", "Reset"="Full Reset", "Type of reset"=w40, "error in (no error)"=w35, "VISA Timeout Value"=u32 10000) -> ("VISA Resource Name out"=w34:refnum<visa-resource-name>, "error out"=w2:errorcluster)
  n10 = Spreadsheet String To Array(delimiter (Tab)="\r\n", format string="%s", spreadsheet string="Program", array type (2D Dbl)="") -> (array=w14:string[][])
  n11 = Array Size(array=w14) -> (size(s)=w18:i32[])
  n12 = String To Path(string=w4) -> (path=w3:path)
  n13 = Write to Text File(file (use dialog)=w3, text=w23, error in=w2) -> (error out=w1:errorcluster)  [unwired: 1 in, 2 out]
  n14 = Index Array(array=w18, index=0) -> (element=w16:i32)
  n15 = for {
    N: w16 -> [w94]
    tunnel: "SMU4" -> [w136]
    shift-left: "Source/Drain Range" -> [w141]
    shift-right: [w137] -> _
    shift-left: "Source/Drain\nRange mode" -> [w142]
    shift-right: [w138] -> _
    shift-left: "Gate Range" -> [w143]
    shift-right: [w139] -> _
    shift-left: "Gate Range\nmode" -> [w144]
    shift-right: [w140] -> _
    shift-left: "Gate: Compliance" -> [w153]
    shift-right: [w149] -> _
    shift-left: "Drain: Compliance" -> [w154]
    shift-right: [w150] -> _
    shift-left: w33 -> [w155]
    shift-right: [w151] -> _
    shift-left: w1 -> [w156]
    shift-right: [w102] -> w9
    shift-left: w34 -> [w157]
    shift-right: [w152] -> _
    shift-left: w5 -> [w158]
    shift-right: [w53] -> _
    tunnel: "Panel Controls 2" -> [w135]
    shift-right: [w106] -> _
    shift-left: _ -> [w134]
    shift-right: [w55] -> _
    shift-left: _ -> [w130]
    tunnel: w14 -> [w129] mode=indexing
    shift-right: [w100] -> _
    shift-left: _ -> [w101]
    shift-right: [w83] -> _
    shift-left: _ -> [w86]
    shift-right: [w56] -> _
    shift-left: _ -> [w76]
    shift-right: [w75] -> _
    shift-left: _ -> [w74]
    shift-right: [w73] -> _
    shift-left: _ -> [w72]
    shift-right: [w50] -> _
    shift-left: _ -> [w51]
    i -> [w89]
    w57 = "Time /s" ("element")
    # "Time array for absolute plunger position"
    # "Valve position"
    # "Valve position"
    # "Pump status"
    # "Absolute plunger position"
    # "Serial port output"
    # "Save serial output log in file."
    # "For loop counter"
    # "<-----Equivalent to the 4155C \"Write\" subvi.----->"
    # "Headers"
    # "Save transfer curves in file."
    # "Filepath and name"
    # "Save time-dependent data."
    # "Use the time offset if your measurements do not start at t=0."
    # "Time for Idmax-Idmin"
    # "Rest of elements of command"
    # "Id min"
    # "Id max"
    # "Limit of command arguments (array columns). Raise if needed."
    # "First element of command\n(case select)"
    n16 = Add(x=w94, y=1) -> (x+y=→"Total lines":i32)
    n17 = Add(x=w89, y=1) -> (x+y=→"Line running":i32)
    n18 = Index Array(array=w129, index=0 ("line index")) -> (element=w124:string)
    "Command running:" <- w124
    n19 = Spreadsheet String To Array(delimiter (Tab)=" ", format string="%s", spreadsheet string=w124, array type (2D Dbl)=string[] []) -> (array=w121:string[])
    n20 = control-ref of="Interrupt run"() -> (w148:refnum<vi>)
    n21 = Delete From Array(array=w121, index=0) -> (deleted portion=w122:string, array with subset deleted=w120:string[])  [unwired: 1 in]
    n22 = call "Elapsed Time"("Reset"="Reset", "Auto Reset"="Auto Reset") -> ("Elapsed Time (s)"=w131:dbl)  [unwired: 10 in, 7 out]
    n23 = case shown="0, Default" "Units" {
      tunnel: ["_sec" "_min" "_h"] -> w132
      tunnel: [w159 w163 w166] -> w96
      tunnel: w131 -> [w159 w162 w167]
      frame 0, Default {
      }
      frame 1 {
        n24 = Divide(x=w162, y=60.0) -> (x/y=w163:dbl)
      }
      frame 2 {
        n25 = Divide(x=w167, y=3600.0) -> (x/y=w166:dbl)
      }
    }
    n26 = Add(x=w96, y="Time Offset") -> (x+y=w95:dbl)
    n27 = To Long Integer(number=w95) -> (32bit integer=w52:i32)
    "Elapsed Time" <- w52
    n28 = case shown="\"pump\"" w122 {
      tunnel: w120 -> [w191 w216 w240 w321 w391 w466 w547 w623 w667 w699 w732 w763 w790 w810 _ _ w932 w999 _ w1076 w1126 w1174 w1250 w1318 w1344 w1398]
      tunnel: w158 -> [w186 w212 w238 w328 w398 w474 w554 w631 w656 w688 w724 w756 w784 w803 w828 w876 w910 w981 w1018 w1063 w1113 w1162 w1244 w1314 w1346 w1400]
      tunnel: w157 -> [w185 w211 w229 w299 w382 w443 w523 w599 w657 w689 w725 w757 w785 w804 w833 w878 w938 w1005 w1022 w1082 w1132 w1180 w1256 w1272 w1350 w1404]
      tunnel: w156 -> [w184 w210 w228 w298 w381 w442 w520 w596 w658 w690 w726 w758 w786 w805 w832 w849 w937 w1004 w1021 w1081 w1131 w1179 w1255 w1271 w1349 w1403]
      tunnel: w155 -> [w183 w209 w237 w324 w357 w470 w550 w627 w666 w698 w723 w755 w783 w802 w831 w873 w901 w973 w1027 w1056 w1106 w1155 w1243 w1313 w1351 w1405]
      tunnel: w154 -> [w182 w208 w236 w326 w396 w472 w552 w629 w665 w697 w731 w762 w789 w809 w830 w858 w936 w1003 w1030 w1080 w1130 w1178 w1254 w1322 w1352 w1406]
      tunnel: w153 -> [w181 w207 w235 w325 w395 w471 w551 w628 w664 w696 w730 w761 w788 w808 w829 w859 w911 w982 w1029 w1064 w1114 w1163 w1245 w1315 w1354 w1407]
      tunnel: [w185 w211 w227 w323 w393 w468 w549 w625 w657 w689 w725 w757 w785 w804 w833 w878 w902 w955 w1020 w1057 w1107 w1156 w1196 w1274 w1350 w1404] -> w152
      tunnel: [w184 w210 w226 w322 w392 w467 w548 w624 w658 w690 w726 w758 w786 w805 w832 w848 w912 w956 w1019 w1065 w1115 w1164 w1195 w1273 w1348 w1402] -> w78
      tunnel: [w183 w209 w237 w324 w353 w470 w550 w627 w659 w691 w723 w755 w783 w802 w831 w873 w901 w973 w1027 w1056 w1106 w1155 w1243 w1313 w1351 w1405] -> w151
      tunnel: [w182 w208 w236 w326 w396 w472 w552 w629 w665 w697 w731 w762 w789 w809 w830 w858 w936 w1003 w1030 w1080 w1130 w1178 w1254 w1322 w1352 w1406] -> w150
      tunnel: [w181 w207 w235 w325 w395 w471 w551 w628 w664 w696 w730 w761 w788 w808 w829 w859 w911 w982 w1029 w1064 w1114 w1163 w1245 w1315 w1354 w1407] -> w149
      tunnel: [w186 w212 w238 w328 w398 w474 w554 w631 w656 w688 w724 w756 w784 w803 w828 w876 w910 w981 w1018 w1063 w1113 w1162 w1244 w1314 w1346 w1400] -> w53
      tunnel: w148 -> [_ _ _ w331 w402 w479 w558 w635 _ _ _ _ _ _ _ _ w907 w978 _ w1062 w1112 w1161 w1216 w1290 _ _]
      tunnel: "Gate" -> [_ _ _ w308 w385 w453 w534 w610 _ _ _ _ _ _ _ _ _ _ _ _ _ _ _ _ _ _]
      tunnel: "Drain 2" -> [_ _ _ w307 w384 w452 w533 w609 _ _ _ _ _ _ _ _ _ _ _ _ _ _ _ _ _ _]
      tunnel: "Panel Controls" -> [_ _ _ _ _ w451 w532 w608 _ _ _ _ _ _ _ _ _ _ _ _ _ _ _ _ _ _]
      tunnel: w144 -> [w180 w206 w234 w292 w375 w436 w518 w594 w663 w695 _ w754 w782 w801 w827 w860 w897 w969 w1023 w1052 w1102 w1151 w1239 w1309 w1355 w1408]
      tunnel: w143 -> [w179 w205 w233 w291 w374 w435 w517 w593 w662 w694 w729 _ w773 w807 w826 w861 w898 w970 w1024 w1053 w1103 w1152 w1240 w1310 w1356 w1409]
      tunnel: w142 -> [w178 w204 w232 w290 w373 w434 w516 w592 w661 w693 w728 w760 w787 _ w825 w862 w899 w971 w1025 w1054 w1104 w1153 w1241 w1311 w1357 w1410]
      tunnel: w141 -> [w177 w203 w231 w289 w372 w433 w519 w595 w660 w692 w727 w759 _ w806 w824 w863 w900 w972 w1026 w1055 w1105 w1154 w1242 w1312 w1358 w1411]
      tunnel: [w180 w206 w234 w292 w375 w436 w518 w594 w663 w695 w722 w754 w782 w801 w827 w860 w897 w969 w1023 w1052 w1102 w1151 w1239 w1309 w1355 w1408] -> w140
      tunnel: [w179 w205 w233 w291 w374 w435 w517 w593 w662 w694 w729 w746 w773 w807 w826 w861 w898 w970 w1024 w1053 w1103 w1152 w1240 w1310 w1356 w1409] -> w139
      tunnel: [w178 w204 w232 w290 w373 w434 w516 w592 w661 w693 w728 w760 w787 w800 w825 w862 w899 w971 w1025 w1054 w1104 w1153 w1241 w1311 w1357 w1410] -> w138
      tunnel: [w177 w203 w231 w289 w372 w433 w519 w595 w660 w692 w727 w759 w774 w806 w824 w863 w900 w972 w1026 w1055 w1105 w1154 w1242 w1312 w1358 w1411] -> w137
      tunnel: w136 -> [_ _ _ w284 w369 _ w512 _ _ _ _ _ _ _ _ _ _ _ _ _ _ _ _ _ _ _]
      tunnel: w135 -> [_ _ _ w282 w368 _ _ _ _ _ _ _ _ _ _ _ _ _ _ _ _ _ _ _ _ _]
      tunnel: [w176 w199 w224 w259 w345 w423 w509 w581 w655 w686 w721 w745 w772 w799 w823 w844 w889 w953 w1017 w1041 w1095 w1145 w1193 w1267 w1347 w1401] -> w106
      tunnel: w134 -> [w176 w199 w224 w273 w345 w423 w509 w581 w655 w686 w721 w745 w772 w799 w823 w844 w889 w953 w1017 w1041 w1095 w1145 w1193 w1267 w1347 w1401]
      tunnel: w95 -> [_ _ _ w269 w342 w421 w506 w578 _ _ _ _ _ _ _ w842 w887 w950 _ w1038 w1092 w1142 w1190 w1263 _ _]
      tunnel: w132 -> [_ _ _ w266 w341 w419 w505 w577 _ _ _ _ _ _ _ w840 w885 w949 _ w1037 w1091 w1141 w1189 w1264 _ w1369]
      tunnel: w52 -> [_ _ _ w260 _ _ _ _ _ _ _ _ _ _ _ _ _ _ _ _ _ _ _ _ _ w1372]
      tunnel: [w175 w198 w223 w257 w344 w422 w508 w580 w654 w685 w720 w744 w771 w798 w822 w843 w888 w952 w1016 w1040 w1094 w1144 w1192 w1266 w1353 w1381] -> w55
      tunnel: w130 -> [w175 w198 w223 w265 w344 w422 w508 w580 w654 w685 w720 w744 w771 w798 w822 w843 w888 w952 w1016 w1040 w1094 w1144 w1192 w1266 w1353 w1381]
      tunnel: [w174 w197 w222 w255 w340 w418 w504 w576 w653 w684 w719 w743 w770 w797 w821 w839 w884 w948 w1015 w1036 w1090 w1140 w1188 w1262 w1342 w1397] -> w100
      tunnel: w101 -> [w174 w197 w222 w254 w340 w418 w504 w576 w653 w684 w719 w743 w770 w797 w821 w839 w884 w948 w1015 w1036 w1090 w1140 w1188 w1262 w1342 w1397]
      tunnel: [w173 w196 w221 w247 w339 w417 w494 w575 w652 w683 w718 w742 w769 w796 w820 w838 w883 w947 w1014 w1035 w1089 w1139 w1187 w1261 w1341 w1396] -> w83
      tunnel: w86 -> [w173 w196 w221 w247 w339 w417 w494 w575 w652 w683 w718 w742 w769 w796 w820 w838 w883 w947 w1014 w1035 w1089 w1139 w1187 w1261 w1340 w1370]
      tunnel: [w172 w195 w220 w246 w338 w416 w493 w574 w651 w682 w717 w741 w768 w795 w819 w837 w882 w946 w1013 w1034 w1088 w1138 w1186 w1260 w1326 w1383] -> w56
      tunnel: w76 -> [w172 w195 w220 w246 w338 w416 w493 w574 w651 w682 w717 w741 w768 w795 w819 w837 w882 w946 w1013 w1034 w1088 w1138 w1186 w1260 w1326 w1382]
      tunnel: [w171 w194 w219 w245 w337 w415 w492 w573 w650 w681 w716 w740 w767 w794 w818 w836 w881 w945 w1012 w1033 w1087 w1137 w1185 w1259 w1325 w1365] -> w75
      tunnel: w74 -> [w171 w194 w219 w245 w337 w415 w492 w573 w650 w681 w716 w740 w767 w794 w818 w836 w881 w945 w1012 w1033 w1087 w1137 w1185 w1259 w1325 w1363]
      tunnel: [w170 w193 w218 w244 w336 w414 w491 w572 w649 w680 w715 w739 w766 w793 w817 w835 w880 w944 w1011 w1032 w1086 w1136 w1184 w1258 w1324 w1362] -> w73
      tunnel: w72 -> [w170 w193 w218 w244 w336 w414 w491 w572 w649 w680 w715 w739 w766 w793 w817 w835 w880 w944 w1011 w1032 w1086 w1136 w1184 w1258 w1324 w1373]
      tunnel: w52 -> [_ _ _ _ _ _ _ _ _ _ _ _ _ _ _ _ _ _ _ _ _ _ _ _ _ w1361]
      tunnel: w51 -> [w169 w192 w217 w243 w335 w413 w490 w571 w648 w679 w714 w738 w765 w792 w816 w834 w879 w943 w1010 w1031 w1085 w1135 w1183 w1257 w1323 w1360]
      tunnel: [w169 w192 w217 w243 w335 w413 w490 w571 w648 w679 w714 w738 w765 w792 w816 w834 w879 w943 w1010 w1031 w1085 w1135 w1183 w1257 w1323 w1359] -> w50
      frame "wait" {
        n29 = Index Array(array=w191, index=0 ("Index")) -> (element=w189:string)
        n30 = Decimal String To Number(string=w189, default (0L)=u32 0) -> (number=w188:u32)  [unwired: 1 in, 1 out]
        n31 = Wait (ms)(milliseconds to wait=w188) -> ()  [unwired: 1 out]
      }
      frame "wait-min" {
        n32 = Index Array(array=w216, index=0 ("Index")) -> (element=w214:string)
        n33 = Decimal String To Number(string=w214, default (0L)=u32 0) -> (number=w202:u32)  [unwired: 1 in, 1 out]
        n34 = Multiply(x=w202, y=u32 60000) -> (x*y=w201:u32)
        n35 = Wait (ms)(milliseconds to wait=w201) -> ()  [unwired: 1 out]
      }
      frame "standby" {
        n36 = Index Array(array=w240, index=0 ("Index")) -> (element=w230:string)
        n37 = case shown="\"on\"" w230 {
          tunnel: [":PAGE:SCON:STAN 0" ":PAGE:SCON:STAN 1"] -> w225
          frame "off", Default {
          }
          frame "on" {
          }
        }
        n38 = VISA Write(VISA resource name=w229, write buffer=w225, error in (no error)=w228) -> (VISA resource name out=w227:refnum<visa-resource-name>, error out=w226:errorcluster)  [unwired: 1 out]
      }
      frame "transfer" {
        # "Don't connect the error lines\nof the two Split blocks!"
        # "Adjusts graph colors."
        # "Time array"
        n39 = Bundle By Name(cluster=w282, "Emergency Stop"=w331) -> (w283:T2)
        n40 = Number To Decimal String(number=w269) -> (decimal integer string=w268:string)  [unwired: 1 in]
        n41 = Delete From Array(array=w321, index=0 ("Index")) -> (deleted portion=w319:string, array with subset deleted=w318:string[])  [unwired: 1 in]
        n42 = Concatenate Strings(w328, "Prefix (transfer)", w268, w266, "Suffix (transfer)") -> (w330:string)
        n43 = VISA Write(VISA resource name=w299, write buffer=":PAGE:CHAN:MODE SWE;" ("write buffer (\"\")"), error in (no error)=w298) -> (VISA resource name out=w296:refnum<visa-resource-name>, error out=w297:errorcluster)  [unwired: 1 out]
        n44 = case shown="\"d\", Default" w319 {
          tunnel: [w333 w334] -> w317
          frame "s" {
            w333 = u16 0 items=["Single", "Double"] ("sweep mode")
          }
          frame "d", Default {
            w334 = u16 1 items=["Single", "Double"] ("sweep mode")
          }
        }
        n45 = String To Path(string=w330) -> (path=w327:path)
        n46 = Fract/Exp String To Number(string=w318) -> (number=w303:dbl[])  [unwired: 3 in, 1 out]
        n47 = Index Array(array=w303, index #1=0 ("Index")) -> (element #1=w316:dbl, element #2=w315:dbl, element #3=w314:dbl)  [unwired: 2 in]
        n48 = Delete From Array(array=w303, length=3 ("Length"), index=0 ("Index")) -> (array with subset deleted=w301:dbl[])  [unwired: 1 out]
        n49 = Build Array (concatenate)(w265, w260) -> (w257:i32[])
        n50 = Bundle By Name(cluster=w308, "Gate Start"=w316, "Gate Stop"=w315, "Gate Step (linear only)"=w314, "Gate Compliance"=w325, "Range mode"=w292, "Range"=w291) -> (w293:T4)
        n51 = call "4155C Split array.vi"("X data in"=w257, "Y1 data in"=w254) -> ("Array of clusters"=w258:cluster{"Y data in":dbl[], "X data in":dbl[]}[])  [unwired: 5 in, 1 out]
        n52 = local write "Id min vs time"(w258) -> ()
        n53 = Index Array(array=w301, index #1=0 ("Index")) -> (element #1=w311:dbl, element #2=w310:dbl, element #3=w309:dbl)  [unwired: 2 in]
        n54 = call <vilib>:"compatOverwrite.vi"("overwrite (F)"=TRUE) -> ("overwrite?"=w281:T7)
        n55 = control-ref of="I vs Vg"() -> (w270:refnum<vi>)
        n56 = Bundle By Name(cluster=w307, "Drain Start"=w311, "Drain Stop"=w310, "Drain Step"=w309, "Drain Compliance"=w326, "Range mode"=w290, "Range"=w289) -> (w294:T5)
        n57 = call "4155C Transfer.vi"("VISA resource name in"=w296, "Gate"=w293, "Drain"=w294, "Timings"=w324, "error in (no error)"=w297, "SMU4"=w284, "sweep mode"=w317, "Panel Controls"=w283) -> ("VG"=w274:dbl[], "Outparams"=w288:T8, "VISA Resource Name out"=w323:refnum<visa-resource-name>, "IS"=w275:dbl[], "ID"=w280:dbl[], "IG"=w276:dbl[], "error out"=w261:errorcluster, "SMU4"=w285:dbl[])  [unwired: 12 in]
        n58 = Unbundle By Name(w288) -> ("V2 Step"=w287:dbl, "V2 Start"=w286:dbl, "Number of points"=w271:i32)
        n59 = call "4155C Split array.vi"("Number of VAR2 steps"=w271, "Y2 data in"=w280, "X data in"=w274, "Y1 data in"=w275, "Y3 data in"=w276, "error in (no error)"=w261) -> ("Array of clusters"=w264:cluster{"Y data in":dbl[], "X data in":dbl[]}[], "error out"=w262:errorcluster)  [unwired: 1 in]
        n60 = local write "I vs Vg"(w264) -> ()
        n61 = Absolute Value(x=w275) -> (abs(x)=w279:dbl[])
        n62 = Array Max & Min(array=w275) -> (max value=w277:dbl)  [unwired: 3 out]
        n63 = Array Max & Min(array=w276) -> (max value=w278:dbl)  [unwired: 3 out]
        n64 = local write "Is"(w277) -> ()
        n65 = Array Max & Min(array=w279) -> (max value=w272:dbl, min value=w256:dbl)  [unwired: 2 out]
        n66 = local write "Ig"(w278) -> ()
        n67 = Build Array (concatenate)(w273, w272) -> (w259:dbl[])
        n68 = call "4155C Split array.vi"("X data in"=w257, "Y1 data in"=w259) -> ("Array of clusters"=w263:cluster{"Y data in":dbl[], "X data in":dbl[]}[])  [unwired: 5 in, 1 out]
        n69 = local write "Id max vs time"(w263) -> ()
        n70 = local write "Id"(w272) -> ()
        n71 = Open/Create/Replace File(file path (use dialog)=w327, error in=w262, operation (0:open)=w281) -> (refnum out=w252:refnum<file>, error out=w250:errorcluster)  [unwired: 3 in, 1 out]
        n72 = call "4155C Make Big 2d array.vi"("1D Var1"=w274, "1d IS"=w275, "1d ID"=w280, "1d IG"=w276, "1d SMU4"=w285, "SMU4"=w284, "VAR2 START"=w286, "Number of VAR2 steps"=w271, "VAR2 STEP"=w287, "VAR1 Name"="Vg", "Decimal places in header"=i8 1, "VAR2 Name"="Vd") -> ("Header array"=w253:string[], "Data array"=w251:dbl[][])  [unwired: 14 in]
        n73 = call "4155C Config Chart Colours.vi"("Numeric"=w271, "XY Graph 2"=w270) -> ()  [unwired: 6 in]
        n74 = call "4155C Write array to file.vi"("Byte Stream File Refnum"=w252, "Header"=w253, "Data Array"=w251, "error in (no error)"=w250) -> ("dup refnum"=w249:refnum<file>, "error out"=w248:errorcluster)  [unwired: 1 in]
        n75 = Build Array (concatenate)(w254, w256) -> (w255:dbl[])
        n76 = Close File(refnum=w249, error in=w248) -> (error out=w322:errorcluster)  [unwired: 1 out]
      }
      frame "pulsedstressV" {
        w351 = 0
        n77 = Number To Decimal String(number=w342) -> (decimal integer string=w399:string)  [unwired: 1 in]
        n78 = Delete From Array(array=w391, index=0 ("Index")) -> (deleted portion=w389:string, array with subset deleted=w388:string[])  [unwired: 1 in]
        n79 = Bundle By Name(cluster=w368, "Emergency Stop"=w402) -> (w370:T2)
        n80 = VISA Write(VISA resource name=w382, write buffer=":PAGE:CHAN:MODE SWE;" ("write buffer (\"\")"), error in (no error)=w381) -> (VISA resource name out=w379:refnum<visa-resource-name>, error out=w380:errorcluster)  [unwired: 1 out]
        n81 = Concatenate Strings(w398, "-pulsedstressV-" ("Substring"), w399, w341, ".txt" ("Substring")) -> (w401:string)
        n82 = case shown="\"d\", Default" w389 {
          tunnel: [w411 w412] -> w387
          frame "s" {
            w411 = u16 0 items=["Single", "Double"] ("sweep mode")
          }
          frame "d", Default {
            w412 = u16 1 items=["Single", "Double"] ("sweep mode")
          }
        }
        n83 = Fract/Exp String To Number(string=w388) -> (number=w383:dbl[])  [unwired: 3 in, 1 out]
        n84 = String To Path(string=w401) -> (path=w397:path)
        n85 = Index Array(array=w383, index #1=0 ("Index")) -> (element #1=w360:dbl, element #2=w359:dbl, element #3=w356:dbl, element #4=w355:dbl, element #5=w354:dbl, element #6=w358:dbl)  [unwired: 5 in]
        n86 = Bundle By Name(cluster=w357, "Pulse period"=w355, "Base voltage"=w356, "Pulse width"=w354) -> (w353:T6)
        n87 = Unbundle By Name(w353) -> ("Pulse period"=w361:dbl)
        n88 = Bundle By Name(cluster=w385, "Gate Start"=w359, "Gate Stop"=w360, "Gate Step (linear only)"=0, "Gate Compliance"=w395, "Range mode"=w375, "Range"=w374) -> (w376:T4)
        n89 = call <vilib>:"compatOverwrite.vi"("overwrite (F)"=TRUE) -> ("overwrite?"=w346:T7)
        n90 = Bundle By Name(cluster=w384, "Drain Start"=w358, "Drain Stop"=w351, "Drain Step"=w351, "Drain Compliance"=w396, "Range mode"=w373, "Range"=w372) -> (w377:T5)
        n91 = call "4155C PulsedStressV.vi"("VISA resource name in"=w379, "sweep mode"=w387, "Panel Controls"=w370, "Gate"=w376, "Drain"=w377, "Timings"=w353, "error in (no error)"=w380, "SMU4"=w369) -> ("VISA Resource Name out"=w393:refnum<visa-resource-name>, "ID"=w349:dbl[], "IG"=w347:dbl[], "Outparams"=w371:T8, "error out"=w394:errorcluster)  [unwired: 3 in]
        n92 = Unbundle By Name(w371) -> ("Number of points"=w348:i32)  [unwired: 2 out]
        n93 = for {
          N: w348 -> [_]
          tunnel: [w408] -> w350 mode=indexing
          tunnel: w361 -> [w410]
          i -> [w409]
          n94 = Multiply(x=w410, y=w409) -> (x*y=w408:dbl)
        }
        n95 = Insert Into Array(array=dbl[][] [] ("Input Array"), new element=w350) -> (w362:dbl[][])  [unwired: 2 in]
        n96 = Insert Into Array(array=w362, new element=w349) -> (w367:dbl[][])  [unwired: 2 in]
        n97 = Insert Into Array(array=w367, new element=w347) -> (w366:dbl[][])  [unwired: 2 in]
        n98 = Transpose 2D Array(2D array=w366) -> (transposed array=w365:dbl[][])
        n99 = Open/Create/Replace File(file path (use dialog)=w397, error in=w394, operation (0:open)=w346) -> (refnum out=w405:refnum<file>, error out=w406:errorcluster)  [unwired: 3 in, 1 out]
        n100 = call "4155C Write array to file.vi"("Byte Stream File Refnum"=w405, "Header"=string[] ["Time /s", "Id /A", "Ig /A"], "Data Array"=w365, "error in (no error)"=w406) -> ("dup refnum"=w403:refnum<file>, "error out"=w404:errorcluster)  [unwired: 1 in]
        n101 = Close File(refnum=w403, error in=w404) -> (error out=w392:errorcluster)  [unwired: 1 out]
      }
      frame "transfer-fpp" {
        n102 = Number To Decimal String(number=w421) -> (decimal integer string=w475:string)  [unwired: 1 in]
        n103 = Bundle By Name(cluster=w451, "Emergency Stop"=w479) -> (w487:T1)
        n104 = Delete From Array(array=w466, index=0 ("Index")) -> (deleted portion=w464:string, array with subset deleted=w463:string[])  [unwired: 1 in]
        n105 = Concatenate Strings(w474, "-transferfpp-" ("Substring"), w475, w419, ".txt" ("Substring")) -> (w477:string)
        n106 = VISA Write(VISA resource name=w443, write buffer=":PAGE:CHAN:MODE SWE;" ("write buffer (\"\")"), error in (no error)=w442) -> (VISA resource name out=w440:refnum<visa-resource-name>, error out=w441:errorcluster)  [unwired: 1 out]
        n107 = case shown="\"d\", Default" w464 {
          tunnel: [w488 w489] -> w462
          frame "s" {
            w488 = u16 0 items=["Single", "Double"] ("sweep mode")
          }
          frame "d", Default {
            w489 = u16 1 items=["Single", "Double"] ("sweep mode")
          }
        }
        n108 = Fract/Exp String To Number(string=w463) -> (number=w447:dbl[])  [unwired: 3 in, 1 out]
        n109 = String To Path(string=w477) -> (path=w473:path)
        n110 = Index Array(array=w447, index #1=0 ("Index")) -> (element #1=w461:dbl, element #2=w460:dbl, element #3=w459:dbl)  [unwired: 2 in]
        n111 = Delete From Array(array=w447, length=3 ("Length"), index=0 ("Index")) -> (array with subset deleted=w445:dbl[])  [unwired: 1 out]
        n112 = Bundle By Name(cluster=w453, "Gate Start"=w461, "Gate Stop"=w460, "Gate Step (linear only)"=w459, "Gate Compliance"=w471, "Range mode"=w436, "Range"=w435) -> (w437:T4)
        n113 = Index Array(array=w445, index #1=0 ("Index")) -> (element #1=w456:dbl, element #2=w455:dbl, element #3=w454:dbl)  [unwired: 2 in]
        n114 = call <vilib>:"compatOverwrite.vi"("overwrite (F)"=TRUE) -> ("overwrite?"=w424:T7)
        n115 = Bundle By Name(cluster=w452, "Drain Start"=w456, "Drain Stop"=w455, "Drain Step"=w454, "Drain Compliance"=w472, "Range mode"=w434, "Range"=w433) -> (w438:T5)
        n116 = call "4155C Transfer-FPP.vi"("VISA resource name in"=w440, "Gate"=w437, "Drain"=w438, "Timings"=w470, "error in (no error)"=w441, "sweep mode"=w462, "Panel Controls"=w487) -> ("VG"=w478:dbl[], "Outparams"=w432:T8, "VISA Resource Name out"=w468:refnum<visa-resource-name>, "Vprobe2"=w428:dbl[], "ID"=w427:dbl[], "IG"=w426:dbl[], "Vprobe1"=w425:dbl[], "error out"=w469:errorcluster)  [unwired: 13 in]
        n117 = Unbundle By Name(w432) -> ("V2 Step"=w431:dbl, "V2 Start"=w430:dbl, "Number of points"=w429:i32)
        n118 = Open/Create/Replace File(file path (use dialog)=w473, error in=w469, operation (0:open)=w424) -> (refnum out=w484:refnum<file>, error out=w485:errorcluster)  [unwired: 3 in, 1 out]
        n119 = call "4155C Make Big 2d array FPP.vi"("1D Var1"=w478, "1d ID"=w427, "1d Vp2"=w428, "1d IG"=w426, "1d Vp1"=w425, "VAR2 START"=w430, "Number of VAR2 steps"=w429, "VAR2 STEP"=w431, "VAR1 Name"="Vg", "Decimal places in header"=i8 1, "VAR2 Name"="Vd") -> ("Header array"=w480:string[], "Data array"=w481:dbl[][])  [unwired: 15 in]
        n120 = call "4155C Write array to file.vi"("Byte Stream File Refnum"=w484, "Header"=w480, "Data Array"=w481, "error in (no error)"=w485) -> ("dup refnum"=w482:refnum<file>, "error out"=w483:errorcluster)  [unwired: 1 in]
        n121 = Close File(refnum=w482, error in=w483) -> (error out=w467:errorcluster)  [unwired: 1 out]
      }
      frame "output" {
        n122 = Number To Decimal String(number=w506) -> (decimal integer string=w555:string)  [unwired: 1 in]
        n123 = Bundle By Name(cluster=w532, "Emergency Stop"=w558) -> (w568:T1)
        n124 = Delete From Array(array=w547, index=0 ("Index")) -> (deleted portion=w545:string, array with subset deleted=w544:string[])  [unwired: 1 in]
        n125 = Concatenate Strings(w554, "Prefix (output)", w555, w505, "Suffix (output)") -> (w557:string)
        n126 = VISA Write(VISA resource name=w523, write buffer=":PAGE:CHAN:MODE SWE;" ("write buffer (\"\")"), error in (no error)=w520) -> (VISA resource name out=w522:refnum<visa-resource-name>, error out=w521:errorcluster)  [unwired: 1 out]
        n127 = case shown="\"d\", Default" w545 {
          tunnel: [w569 w570] -> w543
          frame "s" {
            w569 = u16 0 items=["Single", "Double"] ("sweep mode")
          }
          frame "d", Default {
            w570 = u16 1 items=["Single", "Double"] ("sweep mode")
          }
        }
        n128 = Fract/Exp String To Number(string=w544) -> (number=w526:dbl[])  [unwired: 3 in, 1 out]
        n129 = String To Path(string=w557) -> (path=w553:path)
        n130 = Index Array(array=w526, index #1=0 ("Index")) -> (element #1=w542:dbl, element #2=w541:dbl, element #3=w540:dbl)  [unwired: 2 in]
        n131 = Delete From Array(array=w526, length=3 ("Length"), index=0 ("Index")) -> (array with subset deleted=w525:dbl[])  [unwired: 1 out]
        n132 = control-ref of="I vs Vd"() -> (w496:refnum<vi>)
        n133 = Bundle By Name(cluster=w534, "Gate Start"=w542, "Gate Stop"=w541, "Gate Step (linear only)"=w540, "Gate Compliance"=w551, "Range mode"=w518, "Range"=w517) -> (w567:T4)
        n134 = Index Array(array=w525, index #1=0 ("Index")) -> (element #1=w537:dbl, element #2=w536:dbl, element #3=w535:dbl)  [unwired: 2 in]
        n135 = call <vilib>:"compatOverwrite.vi"("overwrite (F)"=TRUE) -> ("overwrite?"=w510:T7)
        n136 = Bundle By Name(cluster=w533, "Drain Start"=w537, "Drain Stop"=w536, "Drain Step"=w535, "Drain Compliance"=w552, "Range mode"=w516, "Range"=w519) -> (w566:T5)
        n137 = call "4155C Output.vi"("VISA resource name in"=w522, "Gate"=w567, "Drain"=w566, "Timings"=w550, "error in (no error)"=w521, "SMU4"=w512, "sweep mode"=w543, "Panel controls"=w568) -> ("VD"=w503:dbl[], "Outparams"=w514:T8, "VISA Resource Name out"=w549:refnum<visa-resource-name>, "IS"=w502:dbl[], "ID"=w501:dbl[], "IG"=w500:dbl[], "error out"=w498:errorcluster, "SMU4"=w511:dbl[])  [unwired: 12 in]
        n138 = Unbundle By Name(w514) -> ("V2 Step"=w515:dbl, "V2 Start"=w513:dbl, "Number of points"=w495:i32)
        n139 = call "4155C Split array.vi"("Number of VAR2 steps"=w495, "Y2 data in"=w501, "X data in"=w503, "Y1 data in"=w502, "Y3 data in"=w500, "error in (no error)"=w498) -> ("Array of clusters"=w499:cluster{"Y data in":dbl[], "X data in":dbl[]}[], "error out"=w497:errorcluster)  [unwired: 1 in]
        n140 = local write "I vs Vd"(w499) -> ()
        n141 = call "4155C Config Chart Colours.vi"("Numeric"=w495, "XY Graph 2"=w496) -> ()  [unwired: 6 in]
        n142 = Open/Create/Replace File(file path (use dialog)=w553, error in=w497, operation (0:open)=w510) -> (refnum out=w563:refnum<file>, error out=w564:errorcluster)  [unwired: 3 in, 1 out]
        n143 = call "4155C Make Big 2d array.vi"("1D Var1"=w503, "1d IS"=w502, "1d ID"=w501, "1d IG"=w500, "1d SMU4"=w511, "SMU4"=w512, "VAR2 START"=w513, "Number of VAR2 steps"=w495, "VAR2 STEP"=w515, "VAR1 Name"="Vd", "Decimal places in header"=i8 1, "VAR2 Name"="Vg") -> ("Header array"=w559:string[], "Data array"=w560:dbl[][])  [unwired: 14 in]
        n144 = call "4155C Write array to file.vi"("Byte Stream File Refnum"=w563, "Header"=w559, "Data Array"=w560, "error in (no error)"=w564) -> ("dup refnum"=w561:refnum<file>, "error out"=w562:errorcluster)  [unwired: 1 in]
        n145 = Close File(refnum=w561, error in=w562) -> (error out=w548:errorcluster)  [unwired: 1 out]
      }
      frame "output-fpp" {
        n146 = Number To Decimal String(number=w578) -> (decimal integer string=w632:string)  [unwired: 1 in]
        n147 = Bundle By Name(cluster=w608, "Emergency Stop"=w635) -> (w645:T1)
        n148 = Delete From Array(array=w623, index=0 ("Index")) -> (deleted portion=w621:string, array with subset deleted=w620:string[])  [unwired: 1 in]
        n149 = VISA Write(VISA resource name=w599, write buffer=":PAGE:CHAN:MODE SWE;" ("write buffer (\"\")"), error in (no error)=w596) -> (VISA resource name out=w598:refnum<visa-resource-name>, error out=w597:errorcluster)  [unwired: 1 out]
        n150 = Concatenate Strings(w631, "-outputfpp-" ("Substring"), w632, w577, ".txt" ("Substring")) -> (w634:string)
        n151 = case shown="\"d\", Default" w621 {
          tunnel: [w646 w647] -> w619
          frame "s" {
            w646 = u16 0 items=["Single", "Double"] ("sweep mode")
          }
          frame "d", Default {
            w647 = u16 1 items=["Single", "Double"] ("sweep mode")
          }
        }
        n152 = Fract/Exp String To Number(string=w620) -> (number=w602:dbl[])  [unwired: 3 in, 1 out]
        n153 = String To Path(string=w634) -> (path=w630:path)
        n154 = Index Array(array=w602, index #1=0 ("Index")) -> (element #1=w618:dbl, element #2=w617:dbl, element #3=w616:dbl)  [unwired: 2 in]
        n155 = Delete From Array(array=w602, length=3 ("Length"), index=0 ("Index")) -> (array with subset deleted=w601:dbl[])  [unwired: 1 out]
        n156 = Bundle By Name(cluster=w610, "Gate Start"=w618, "Gate Stop"=w617, "Gate Step (linear only)"=w616, "Gate Compliance"=w628, "Range mode"=w594, "Range"=w593) -> (w644:T4)
        n157 = Index Array(array=w601, index #1=0 ("Index")) -> (element #1=w613:dbl, element #2=w612:dbl, element #3=w611:dbl)  [unwired: 2 in]
        n158 = call <vilib>:"compatOverwrite.vi"("overwrite (F)"=TRUE) -> ("overwrite?"=w582:T7)
        n159 = Bundle By Name(cluster=w609, "Drain Start"=w613, "Drain Stop"=w612, "Drain Step"=w611, "Drain Compliance"=w629, "Range mode"=w592, "Range"=w595) -> (w643:T5)
        n160 = call "4155C Output-FPP.vi"("VISA resource name in"=w598, "Gate"=w644, "Drain"=w643, "Timings"=w627, "error in (no error)"=w597, "sweep mode"=w619, "Panel controls"=w645) -> ("VD"=w587:dbl[], "Outparams"=w590:T8, "VISA Resource Name out"=w625:refnum<visa-resource-name>, "Vprobe2"=w586:dbl[], "ID"=w585:dbl[], "IG"=w584:dbl[], "Vprobe1"=w583:dbl[], "error out"=w626:errorcluster)  [unwired: 13 in]
        n161 = Unbundle By Name(w590) -> ("V2 Step"=w591:dbl, "V2 Start"=w589:dbl, "Number of points"=w588:i32)
        n162 = Open/Create/Replace File(file path (use dialog)=w630, error in=w626, operation (0:open)=w582) -> (refnum out=w640:refnum<file>, error out=w641:errorcluster)  [unwired: 3 in, 1 out]
        n163 = call "4155C Make Big 2d array FPP.vi"("1D Var1"=w587, "1d ID"=w585, "1d Vp2"=w586, "1d IG"=w584, "1d Vp1"=w583, "VAR2 START"=w589, "Number of VAR2 steps"=w588, "VAR2 STEP"=w591, "VAR1 Name"="Vd", "Decimal places in header"=i8 1, "VAR2 Name"="Vg") -> ("Header array"=w636:string[], "Data array"=w637:dbl[][])  [unwired: 15 in]
        n164 = call "4155C Write array to file.vi"("Byte Stream File Refnum"=w640, "Header"=w636, "Data Array"=w637, "error in (no error)"=w641) -> ("dup refnum"=w638:refnum<file>, "error out"=w639:errorcluster)  [unwired: 1 in]
        n165 = Close File(refnum=w638, error in=w639) -> (error out=w624:errorcluster)  [unwired: 1 out]
      }
      frame "itime" {
        n166 = Delete From Array(array=w667, index=0 ("Index")) -> (deleted portion=w668:string)  [unwired: 1 in, 1 out]
        n167 = case shown="\"l\"" w668 {
          tunnel: w666 -> [w672 w674 w677]
          tunnel: [w671 w673 w676] -> w659
          frame "s" {
            w670 = u32 0 items=["short  ", "medium  ", "long  "] ("integration time 2")
            n168 = Bundle By Name(cluster=w672, "integration time"=w670) -> (w671:T6)
          }
          frame "m", Default {
            w675 = u32 1 items=["short  ", "medium  ", "long  "] ("integration time 2")
            n169 = Bundle By Name(cluster=w674, "integration time"=w675) -> (w673:T6)
          }
          frame "l" {
            w678 = u32 2 items=["short  ", "medium  ", "long  "] ("integration time 2")
            n170 = Bundle By Name(cluster=w677, "integration time"=w678) -> (w676:T6)
          }
        }
      }
      frame "pulsed" {
        n171 = Delete From Array(array=w699, index=0 ("Index")) -> (deleted portion=w700:string, array with subset deleted=w687:string[])  [unwired: 1 in]
        n172 = case shown="\"on\", Default" w700 {
          tunnel: w698 -> [w710 w713]
          tunnel: [w709 w712] -> w691
          tunnel: w687 -> [w707 _]
          frame "on", Default {
            w708 = u16 1 items=["Continuous", "Pulsed"] ("sweep method")
            n173 = Fract/Exp String To Number(string=w707) -> (number=w705:dbl[])  [unwired: 3 in, 1 out]
            n174 = Index Array(array=w705, index #1=0 ("Index")) -> (element #1=w704:dbl, element #2=w703:dbl, element #3=w702:dbl)  [unwired: 2 in]
            n175 = Bundle By Name(cluster=w710, "sweep method"=w708, "Pulse period"=w704, "Base voltage"=w703, "Pulse width"=w702) -> (w709:T6)
          }
          frame "off" {
            w711 = u16 0 items=["Continuous", "Pulsed"] ("sweep method")
            n176 = Bundle By Name(cluster=w713, "sweep method"=w711) -> (w712:T6)
          }
        }
      }
      frame "gaterangemode" {
        n177 = Delete From Array(array=w732, index=0 ("Index")) -> (deleted portion=w733:string)  [unwired: 1 in, 1 out]
        n178 = case shown="\"f\"" w733 {
          tunnel: [w735 w736 w737] -> w722
          frame "a", Default {
            w735 = u16 0 items=["Auto", "Limited", "Fixed"] ("Gate Range\nmode 2")
          }
          frame "f" {
            w736 = u16 2 items=["Auto", "Limited", "Fixed"] ("Gate Range\nmode 2")
          }
          frame "l" {
            w737 = u16 1 items=["Auto", "Limited", "Fixed"] ("Gate Range\nmode 2")
          }
        }
      }
      frame "gaterange" {
        (unwired) u8 11 items=["10fA  ", "100fA  ", "1nA  ", "10nA", "100nA", "1uA", "10uA", "100uA", "1mA", "10mA", "100mA", "1A"] ("Gate Range 2")
        n179 = Delete From Array(array=w763, index=0 ("Index")) -> (deleted portion=w753:string)  [unwired: 1 in, 1 out]
        n180 = Scan Value(string=w753, format string="") -> (value=w751:dbl)  [unwired: 1 in, 1 out]
        n181 = Logarithm Base 10(1:w751) -> (0:w750:dbl)
        n182 = Round To Nearest(number=w750) -> (nearest integer value=w749:dbl)
        n183 = Add(x=w749, y=11.0) -> (x+y=w747:dbl)
        n184 = To Unsigned Byte Integer(number=w747) -> (unsigned 8bit integer=w746:u8)
      }
      frame "drainrange" {
        (unwired) u8 11 items=["10fA  ", "100fA  ", "1nA  ", "10nA", "100nA", "1uA", "10uA", "100uA", "1mA", "10mA", "100mA", "1A"] ("Gate Range 2")
        n185 = Delete From Array(array=w790, index=0 ("Index")) -> (deleted portion=w781:string)  [unwired: 1 in, 1 out]
        n186 = Scan Value(string=w781, format string="") -> (value=w779:dbl)  [unwired: 1 in, 1 out]
        n187 = Logarithm Base 10(1:w779) -> (0:w778:dbl)
        n188 = Round To Nearest(number=w778) -> (nearest integer value=w777:dbl)
        n189 = Add(x=w777, y=11.0) -> (x+y=w775:dbl)
        n190 = To Unsigned Byte Integer(number=w775) -> (unsigned 8bit integer=w774:u8)
      }
      frame "drainrangemode" {
        n191 = Delete From Array(array=w810, index=0 ("Index")) -> (deleted portion=w811:string)  [unwired: 1 in, 1 out]
        n192 = case shown="\"f\"" w811 {
          tunnel: [w813 w814 w815] -> w800
          frame "a", Default {
            w813 = u16 0 items=["Auto", "Limited", "Fixed"] ("Gate Range\nmode 2")
          }
          frame "f" {
            w814 = u16 2 items=["Auto", "Limited", "Fixed"] ("Gate Range\nmode 2")
          }
          frame "l" {
            w815 = u16 1 items=["Auto", "Limited", "Fixed"] ("Gate Range\nmode 2")
          }
        }
      }
      frame "Error", Default {
      }
      frame "logfile" {
        n193 = Number To Decimal String(number=w842) -> (decimal integer string=w877:string)  [unwired: 1 in]
        n194 = Concatenate Strings(w876, "logfile" ("Substring"), w877, w840, ".txt" ("Substring")) -> (w874:string)
        n195 = String To Path(string=w874) -> (path=w847:path)
        n196 = Unbundle(w873) -> ("integration time"=w872:u32, "Short/Long integration time"=w871:dbl, "hold time (sec)"=w870:dbl, "delay time (sec)"=w869:dbl, "Step Time (0 disables)"=w868:dbl, "sweep method"=w867:u16, "Pulse period"=w866:dbl, "Base voltage"=w865:dbl, "Pulse width"=w864:dbl)
        n197 = Build Array(w872, w871, w870, w869, w868, w867, w866, w865, w864, w858, w859, w860, w861, w862, w863) -> (w851:dbl[])
        n198 = Insert Into Array(array=dbl[][] [] ("Input Array"), new element=w851) -> (w850:dbl[][])  [unwired: 2 in]
        n199 = call <vilib>:"compatOverwrite.vi"("overwrite (F)"=TRUE) -> ("overwrite?"=w845:T7)
        n200 = Open/Create/Replace File(file path (use dialog)=w847, error in=w849, operation (0:open)=w845) -> (refnum out=w855:refnum<file>, error out=w854:errorcluster)  [unwired: 3 in, 1 out]
        n201 = call "4155C Write array to file.vi"("Byte Stream File Refnum"=w855, "Header"=string[] ["Int Time", "Short/Long Itime", "Hold time", "Delay time", "Step time", "Sweep method", "Pulse period", "Base Voltage", "Pulse width", "Drain compliance", "Gate compliance", "Gate range mode", "Gate range", "S/D range mode", "S/D range"], "Data Array"=w850, "error in (no error)"=w854) -> ("dup refnum"=w857:refnum<file>, "error out"=w856:errorcluster)  [unwired: 1 in]
        n202 = Close File(refnum=w857, error in=w856) -> (error out=w848:errorcluster)  [unwired: 1 out]
      }
      frame "sample" {
        n203 = Number To Decimal String(number=w887) -> (decimal integer string=w935:string)  [unwired: 1 in]
        n204 = Fract/Exp String To Number(string=w932) -> (number=w893:dbl[])  [unwired: 3 in, 1 out]
        n205 = Concatenate Strings(w910, "-sample-" ("Substring"), w935, w885, ".txt" ("Substring")) -> (w933:string)
        n206 = String To Path(string=w933) -> (path=w914:path)
        n207 = Index Array(array=w893, index=0 ("Index")) -> (element=w930:dbl)
        n208 = Index Array(array=w893, index=2 ("Index")) -> (element=w926:dbl)
        n209 = Index Array(array=w893, index=3 ("Index")) -> (element=w895:dbl)
        n210 = Index Array(array=w893, index=4 ("Index")) -> (element=w892:dbl)
        n211 = call "4155C Config Sampling Measurements.vi"("Sampling interval"=w892, "Sample time"=w895, "Display on/off"=TRUE, "Timings"=w901, "Num Points"=w926, "error in (no error)"=w937, "Drain Compliance"=w936, "Gate Compliance"=w911, "VISA session"=w938) -> ("error out"=w939:errorcluster, "dup VISA resource name"=w940:refnum<visa-resource-name>)  [unwired: 1 in]
        n212 = Index Array(array=w893, index=1 ("Index")) -> (element=w927:dbl)
        n213 = call "4155C Take Sample.vi"("Emergency Stop"=w907, "error in (no error)"=w939, "Vd"=w927, "Vg"=w930, "VISA resource name in"=w940) -> ("error out"=w905:errorcluster, "Id"=w942:dbl[], "Ig"=w916:dbl[], "VISA Resource Name out"=w903:refnum<visa-resource-name>, "Is"=w941:dbl[], "Time"=w920:dbl[])  [unwired: 1 in]
        n214 = Insert Into Array(array=dbl[][] [] ("Input Array"), new element=w920) -> (w919:dbl[][])  [unwired: 2 in]
        n215 = Insert Into Array(array=w919, new element=w916) -> (w918:dbl[][])  [unwired: 2 in]
        n216 = Insert Into Array(array=w918, new element=w942) -> (w917:dbl[][])  [unwired: 2 in]
        n217 = VISA Write(VISA resource name=w903, write buffer=":DISP ON" ("write buffer (\"\")"), error in (no error)=w905) -> (VISA resource name out=w902:refnum<visa-resource-name>, error out=w904:errorcluster)  [unwired: 1 out]
        n218 = Insert Into Array(array=w917, new element=w941) -> (w909:dbl[][])  [unwired: 2 in]
        n219 = Transpose 2D Array(2D array=w909) -> (transposed array=w908:dbl[][])
        n220 = call <vilib>:"compatOverwrite.vi"("overwrite (F)"=TRUE) -> ("overwrite?"=w890:T7)
        n221 = Open/Create/Replace File(file path (use dialog)=w914, error in=w904, operation (0:open)=w890) -> (refnum out=w923:refnum<file>, error out=w922:errorcluster)  [unwired: 3 in, 1 out]
        n222 = call "4155C Write array to file.vi"("Byte Stream File Refnum"=w923, "Header"=string[] ["Time /s", "Ig /A", "Id /A", "Is /A"], "Data Array"=w908, "error in (no error)"=w922) -> ("dup refnum"=w925:refnum<file>, "error out"=w924:errorcluster)  [unwired: 1 in]
        n223 = Close File(refnum=w925, error in=w924) -> (error out=w912:errorcluster)  [unwired: 1 out]
      }
      frame "samplei" {
        n224 = Number To Decimal String(number=w950) -> (decimal integer string=w1002:string)  [unwired: 1 in]
        n225 = Fract/Exp String To Number(string=w999) -> (number=w966:dbl[])  [unwired: 3 in, 1 out]
        n226 = Concatenate Strings(w981, "-samplei-" ("Substring"), w1002, w949, ".txt" ("Substring")) -> (w1000:string)
        n227 = String To Path(string=w1000) -> (path=w984:path)
        n228 = Index Array(array=w966, index=4 ("Index")) -> (element=w960:dbl)
        n229 = Index Array(array=w966, index=3 ("Index")) -> (element=w961:dbl)
        n230 = Index Array(array=w966, index=1 ("Index")) -> (element=w963:dbl)
        n231 = Index Array(array=w966, index=0 ("Index")) -> (element=w964:dbl)
        n232 = Index Array(array=w966, index=2 ("Index")) -> (element=w962:dbl)
        n233 = call "4155C Config SamplingI Measurements.vi"("Sample time"=w962, "Display on/off"=TRUE, "Timings"=w973, "Num Points"=w963, "error in (no error)"=w1004, "Sampling interval"=w961, "VISA session"=w1005) -> ("error out"=w1006:errorcluster, "dup VISA resource name"=w1007:refnum<visa-resource-name>)  [unwired: 3 in]
        n234 = call "4155C Take SampleI.vi"("Emergency Stop"=w978, "error in (no error)"=w1006, "Idg 2"=w964, "Vdg compliance 2"=w960, "VISA resource name in"=w1007) -> ("error out"=w976:errorcluster, "Idg"=w1009:dbl[], "Vdg"=w986:dbl[], "VISA Resource Name out"=w974:refnum<visa-resource-name>, "Is"=w1008:dbl[], "Time"=w990:dbl[])  [unwired: 1 in]
        n235 = Insert Into Array(array=dbl[][] [] ("Input Array"), new element=w990) -> (w989:dbl[][])  [unwired: 2 in]
        n236 = Insert Into Array(array=w989, new element=w986) -> (w988:dbl[][])  [unwired: 2 in]
        n237 = Insert Into Array(array=w988, new element=w1009) -> (w987:dbl[][])  [unwired: 2 in]
        n238 = VISA Write(VISA resource name=w974, write buffer=":DISP ON" ("write buffer (\"\")"), error in (no error)=w976) -> (VISA resource name out=w959:refnum<visa-resource-name>, error out=w975:errorcluster)  [unwired: 1 out]
        n239 = Insert Into Array(array=w987, new element=w1008) -> (w980:dbl[][])  [unwired: 2 in]
        n240 = Transpose 2D Array(2D array=w980) -> (transposed array=w979:dbl[][])
        n241 = call <vilib>:"compatOverwrite.vi"("overwrite (F)"=TRUE) -> ("overwrite?"=w954:T7)
        n242 = Open/Create/Replace File(file path (use dialog)=w984, error in=w975, operation (0:open)=w954) -> (refnum out=w993:refnum<file>, error out=w992:errorcluster)  [unwired: 3 in, 1 out]
        n243 = call "4155C Write array to file.vi"("Byte Stream File Refnum"=w993, "Header"=string[] ["Time /s", "Vdg /V", "Idg /A", "Is /A"], "Data Array"=w979, "error in (no error)"=w992) -> ("dup refnum"=w995:refnum<file>, "error out"=w994:errorcluster)  [unwired: 1 in]
        n244 = Close File(refnum=w995, error in=w994) -> (error out=w957:errorcluster)  [unwired: 1 out]
        n245 = VISA Write(VISA resource name=w959, write buffer=";:PAGE:SCON:STAN OFF;:PAGE:CHAN:VSU2:DIS;" ("write buffer (\"\")"), error in (no error)=w957) -> (VISA resource name out=w955:refnum<visa-resource-name>, error out=w956:errorcluster)  [unwired: 1 out]
      }
      frame "#" {
        n246 = VISA Write(VISA resource name=w1022, write buffer=":DISP ON" ("write buffer (\"\")"), error in (no error)=w1021) -> (VISA resource name out=w1020:refnum<visa-resource-name>, error out=w1019:errorcluster)  [unwired: 1 out]
      }
      frame "stressV" {
        n247 = Number To Decimal String(number=w1038) -> (decimal integer string=w1079:string)  [unwired: 1 in]
        n248 = Fract/Exp String To Number(string=w1076) -> (number=w1049:dbl[])  [unwired: 3 in, 1 out]
        n249 = Concatenate Strings(w1063, "-stressV-" ("Substring"), w1079, w1037, ".txt" ("Substring")) -> (w1077:string)
        n250 = String To Path(string=w1077) -> (path=w1067:path)
        n251 = Index Array(array=w1049, index=3 ("Index")) -> (element=w1046:dbl)
        n252 = Index Array(array=w1049, index=1 ("Index")) -> (element=w1044:dbl)
        n253 = Index Array(array=w1049, index=0 ("Index")) -> (element=w1043:dbl)
        n254 = Index Array(array=w1049, index=4 ("Index")) -> (element=w1048:dbl)
        n255 = Index Array(array=w1049, index=2 ("Index")) -> (element=w1045:dbl)
        n256 = call "4155C Config V Stress.vi"("VISA session"=w1082, "ID compliance"=w1046, "VD"=w1044, "VG"=w1043, "IG compliance"=w1045, "error in (no error)"=w1081, "Display on/off"=TRUE) -> ("dup VISA resource name"=w1084:refnum<visa-resource-name>, "error out"=w1083:errorcluster)
        n257 = call "4155C Apply Stress.vi"("error in (no error)"=w1083, "Duration"=w1048, "Emergency Stop"=w1062, "VISA resource name in"=w1084) -> ("error out"=w1060:errorcluster, "VISA Resource Name out"=w1058:refnum<visa-resource-name>)
        n258 = VISA Write(VISA resource name=w1058, write buffer=":DISP ON" ("write buffer (\"\")"), error in (no error)=w1060) -> (VISA resource name out=w1057:refnum<visa-resource-name>, error out=w1059:errorcluster)  [unwired: 1 out]
        n259 = call <vilib>:"compatOverwrite.vi"("overwrite (F)"=TRUE) -> ("overwrite?"=w1042:T7)
        n260 = Open/Create/Replace File(file path (use dialog)=w1067, error in=w1059, operation (0:open)=w1042) -> (refnum out=w1070:refnum<file>, error out=w1069:errorcluster)  [unwired: 3 in, 1 out]
        n261 = call "4155C Write array to file.vi"("Byte Stream File Refnum"=w1070, "Header"=string[] ["V stress completed successfully", ""], "error in (no error)"=w1069) -> ("dup refnum"=w1072:refnum<file>, "error out"=w1071:errorcluster)  [unwired: 2 in]
        n262 = Close File(refnum=w1072, error in=w1071) -> (error out=w1065:errorcluster)  [unwired: 1 out]
      }
      frame "stressI" {
        n263 = Number To Decimal String(number=w1092) -> (decimal integer string=w1129:string)  [unwired: 1 in]
        n264 = Fract/Exp String To Number(string=w1126) -> (number=w1101:dbl[])  [unwired: 3 in, 1 out]
        n265 = Concatenate Strings(w1113, "-stressI-" ("Substring"), w1129, w1091, ".txt" ("Substring")) -> (w1127:string)
        n266 = String To Path(string=w1127) -> (path=w1117:path)
        n267 = Index Array(array=w1101, index=1 ("Index")) -> (element=w1097:dbl)
        n268 = Index Array(array=w1101, index=0 ("Index")) -> (element=w1098:dbl)
        n269 = call "4155C Config I Stress.vi"("VISA session"=w1132, "IDG"=w1098, "VDG compliance"=w1097, "error in (no error)"=w1131, "Display on/off"=TRUE) -> ("dup VISA resource name"=w1134:refnum<visa-resource-name>, "error out"=w1133:errorcluster)
        n270 = Index Array(array=w1101, index=2 ("Index")) -> (element=w1099:dbl)
        n271 = call "4155C Apply Stress.vi"("error in (no error)"=w1133, "Duration"=w1099, "Emergency Stop"=w1112, "VISA resource name in"=w1134) -> ("error out"=w1110:errorcluster, "VISA Resource Name out"=w1108:refnum<visa-resource-name>)
        n272 = VISA Write(VISA resource name=w1108, write buffer=":DISP ON" ("write buffer (\"\")"), error in (no error)=w1110) -> (VISA resource name out=w1107:refnum<visa-resource-name>, error out=w1109:errorcluster)  [unwired: 1 out]
        n273 = call <vilib>:"compatOverwrite.vi"("overwrite (F)"=TRUE) -> ("overwrite?"=w1096:T7)
        n274 = Open/Create/Replace File(file path (use dialog)=w1117, error in=w1109, operation (0:open)=w1096) -> (refnum out=w1120:refnum<file>, error out=w1119:errorcluster)  [unwired: 3 in, 1 out]
        n275 = call "4155C Write array to file.vi"("Byte Stream File Refnum"=w1120, "Header"=string[] ["I stress completed successfully", ""], "error in (no error)"=w1119) -> ("dup refnum"=w1122:refnum<file>, "error out"=w1121:errorcluster)  [unwired: 2 in]
        n276 = Close File(refnum=w1122, error in=w1121) -> (error out=w1115:errorcluster)  [unwired: 1 out]
      }
      frame "vsu2pulse" {
        n277 = Number To Decimal String(number=w1142) -> (decimal integer string=w1177:string)  [unwired: 1 in]
        n278 = Fract/Exp String To Number(string=w1174) -> (number=w1150:dbl[])  [unwired: 3 in, 1 out]
        n279 = Concatenate Strings(w1162, "-vsu2-" ("Substring"), w1177, w1141, ".txt" ("Substring")) -> (w1175:string)
        n280 = String To Path(string=w1175) -> (path=w1166:path)
        n281 = Index Array(array=w1150, index=1 ("Index")) -> (element=w1149:dbl)
        n282 = Index Array(array=w1150, index=0 ("Index")) -> (element=w1147:dbl)
        n283 = call "4155C Config VSU2 Stress.vi"("error in (no error)"=w1179, "VSU2"=w1147, "Display on/off"=TRUE, "VISA session"=w1180) -> ("error out"=w1181:errorcluster, "dup VISA resource name"=w1182:refnum<visa-resource-name>)
        n284 = call "4155C Apply Stress.vi"("error in (no error)"=w1181, "Duration"=w1149, "Emergency Stop"=w1161, "VISA resource name in"=w1182) -> ("error out"=w1159:errorcluster, "VISA Resource Name out"=w1157:refnum<visa-resource-name>)
        n285 = VISA Write(VISA resource name=w1157, write buffer=":DISP ON" ("write buffer (\"\")"), error in (no error)=w1159) -> (VISA resource name out=w1156:refnum<visa-resource-name>, error out=w1158:errorcluster)  [unwired: 1 out]
        n286 = call <vilib>:"compatOverwrite.vi"("overwrite (F)"=TRUE) -> ("overwrite?"=w1146:T7)
        n287 = Open/Create/Replace File(file path (use dialog)=w1166, error in=w1158, operation (0:open)=w1146) -> (refnum out=w1169:refnum<file>, error out=w1168:errorcluster)  [unwired: 3 in, 1 out]
        n288 = call "4155C Write array to file.vi"("Byte Stream File Refnum"=w1169, "Header"=string[] ["VSU2 pulse completed successfully", ""], "error in (no error)"=w1168) -> ("dup refnum"=w1171:refnum<file>, "error out"=w1170:errorcluster)  [unwired: 2 in]
        n289 = Close File(refnum=w1171, error in=w1170) -> (error out=w1164:errorcluster)  [unwired: 1 out]
      }
      frame "sample-fpp" {
        w1201 = string[] ["Time /s", "Id VgVd /A", "Ig VgVd /A", "Vp1 VgVd /V", "Vp2 VgVd /V"] ("Header")
        w1205 = "%d" ("format string")
        n290 = Number To Decimal String(number=w1190) -> (decimal integer string=w1253:string)  [unwired: 1 in]
        n291 = Fract/Exp String To Number(string=w1250) -> (number=w1238:dbl[])  [unwired: 3 in, 1 out]
        n292 = Concatenate Strings(w1244, "-samplefpp-" ("Substring"), w1253, w1189, ".txt" ("Substring")) -> (w1251:string)
        n293 = String To Path(string=w1251) -> (path=w1213:path)
        n294 = Index Array(array=w1238, index=0 ("Index")) -> (element=w1199:dbl)
        n295 = Index Array(array=w1238, index=1 ("Index")) -> (element=w1198:dbl)
        n296 = Index Array(array=w1238, index=2 ("Index")) -> (element=w1246:dbl)
        n297 = Index Array(array=w1238, index=3 ("Index")) -> (element=w1236:dbl)
        n298 = call "4155C Config Sampling Measurements FPP.vi"("VISA session"=w1256, "Num Points"=w1246, "Vg"=w1199, "Display on/off"=TRUE, "Gate Compliance"=w1245, "Drain Compliance"=w1254, "Standby"="Standby", "error in (no error)"=w1255, "Timings"=w1243, "Vd"=w1198, "Sample time"=w1236) -> ("dup VISA resource name"=w1215:refnum<visa-resource-name>, "error out"=w1214:errorcluster)  [unwired: 3 in]
        n299 = Number To Decimal String(number=w1199) -> (decimal integer string=w1225:string)  [unwired: 1 in]
        n300 = call "4155C Take Sample FPP.vi"("VISA resource name in"=w1215, "error in (no error)"=w1214, "Emergency Stop"=w1216) -> ("Time"=w1220:dbl[], "Vp1"=w1230:dbl[], "VISA Resource Name out"=w1196:refnum<visa-resource-name>, "Ig"=w1218:dbl[], "Id"=w1219:dbl[], "Vp2"=w1228:dbl[], "error out"=w1217:errorcluster)  [unwired: 10 in]
        n301 = Insert Into Array(array=dbl[][] [] ("Input Array"), new element=w1220) -> (w1234:dbl[][])  [unwired: 2 in]
        n302 = Number To Decimal String(number=w1198) -> (decimal integer string=w1223:string)  [unwired: 1 in]
        n303 = Insert Into Array(array=w1234, new element=w1219) -> (w1233:dbl[][])  [unwired: 2 in]
        n304 = Concatenate Strings("(Vg = " ("Substring"), w1225, "V, Vd = " ("Substring"), w1223, "V)" ("Substring")) -> (w1221:string)
        n305 = Insert Into Array(array=w1233, new element=w1218) -> (w1232:dbl[][])  [unwired: 2 in]
        n306 = Insert Into Array(array=w1232, new element=w1230) -> (w1229:dbl[][])  [unwired: 2 in]
        n307 = Insert Into Array(array=w1229, new element=w1228) -> (w1197:dbl[][])  [unwired: 2 in]
        n308 = call <vilib>:"compatOverwrite.vi"("overwrite (F)"=TRUE) -> ("overwrite?"=w1194:T7)
        n309 = Open/Create/Replace File(file path (use dialog)=w1213, error in=w1217, operation (0:open)=w1194) -> (refnum out=w1210:refnum<file>, error out=w1211:errorcluster)  [unwired: 3 in, 1 out]
        n310 = Array To Spreadsheet String(array=w1201, 3:w1205) -> (spreadsheet string=w1207:string)  [unwired: 1 in]
        n311 = Transpose 2D Array(2D array=w1197) -> (transposed array=w1227:dbl[][])
        n312 = Search and Replace String(replace all?=TRUE ("replace all? (F)"), input string=w1207, search string="VgVd", replace string=w1221) -> (result string=w1203:string)  [unwired: 4 in, 3 out]
        n313 = Spreadsheet String To Array(format string=w1205, spreadsheet string=w1203, array type (2D Dbl)=w1201) -> (array=w1202:string[])  [unwired: 1 in]
        n314 = call "4155C Write array to file.vi"("Byte Stream File Refnum"=w1210, "Header"=w1202, "Data Array"=w1227, "error in (no error)"=w1211) -> ("dup refnum"=w1208:refnum<file>, "error out"=w1209:errorcluster)  [unwired: 1 in]
        n315 = Close File(refnum=w1208, error in=w1209) -> (error out=w1195:errorcluster)  [unwired: 1 out]
      }
      frame "resample-fpp" {
        w1277 = string[] ["Time /s", "Id VgVd /A", "Ig VgVd /A", "Vp1 VgVd /V", "Vp2 VgVd /V"] ("Header")
        w1281 = "%d" ("format string")
        n316 = Number To Decimal String(number=w1263) -> (decimal integer string=w1321:string)  [unwired: 1 in]
        n317 = Fract/Exp String To Number(string=w1318) -> (number=w1270:dbl[])  [unwired: 3 in, 1 out]
        n318 = Concatenate Strings(w1314, "-resamplefpp-" ("Substring"), w1321, w1264, ".txt" ("Substring")) -> (w1319:string)
        n319 = String To Path(string=w1319) -> (path=w1289:path)
        n320 = Index Array(array=w1270, index=0 ("Index")) -> (element=w1276:dbl)
        n321 = Index Array(array=w1270, index=1 ("Index")) -> (element=w1275:dbl)
        n322 = Number To Decimal String(number=w1276) -> (decimal integer string=w1299:string)  [unwired: 1 in]
        n323 = call "4155C Take Sample FPP.vi"("VISA resource name in"=w1272, "error in (no error)"=w1271, "Emergency Stop"=w1290) -> ("Time"=w1294:dbl[], "Vp1"=w1304:dbl[], "VISA Resource Name out"=w1274:refnum<visa-resource-name>, "Ig"=w1292:dbl[], "Id"=w1293:dbl[], "Vp2"=w1302:dbl[], "error out"=w1291:errorcluster)  [unwired: 10 in]
        n324 = Insert Into Array(array=dbl[][] [] ("Input Array"), new element=w1294) -> (w1308:dbl[][])  [unwired: 2 in]
        n325 = Number To Decimal String(number=w1275) -> (decimal integer string=w1297:string)  [unwired: 1 in]
        n326 = Insert Into Array(array=w1308, new element=w1293) -> (w1307:dbl[][])  [unwired: 2 in]
        n327 = Concatenate Strings("(Vg = " ("Substring"), w1299, "V, Vd = " ("Substring"), w1297, "V)" ("Substring")) -> (w1295:string)
        n328 = Insert Into Array(array=w1307, new element=w1292) -> (w1306:dbl[][])  [unwired: 2 in]
        n329 = Insert Into Array(array=w1306, new element=w1304) -> (w1303:dbl[][])  [unwired: 2 in]
        n330 = Insert Into Array(array=w1303, new element=w1302) -> (w1269:dbl[][])  [unwired: 2 in]
        n331 = call <vilib>:"compatOverwrite.vi"("overwrite (F)"=TRUE) -> ("overwrite?"=w1268:T7)
        n332 = Open/Create/Replace File(file path (use dialog)=w1289, error in=w1291, operation (0:open)=w1268) -> (refnum out=w1286:refnum<file>, error out=w1287:errorcluster)  [unwired: 3 in, 1 out]
        n333 = Array To Spreadsheet String(array=w1277, 3:w1281) -> (spreadsheet string=w1283:string)  [unwired: 1 in]
        n334 = Transpose 2D Array(2D array=w1269) -> (transposed array=w1301:dbl[][])
        n335 = Search and Replace String(replace all?=TRUE ("replace all? (F)"), input string=w1283, search string="VgVd", replace string=w1295) -> (result string=w1279:string)  [unwired: 4 in, 3 out]
        n336 = Spreadsheet String To Array(format string=w1281, spreadsheet string=w1279, array type (2D Dbl)=w1277) -> (array=w1278:string[])  [unwired: 1 in]
        n337 = call "4155C Write array to file.vi"("Byte Stream File Refnum"=w1286, "Header"=w1278, "Data Array"=w1301, "error in (no error)"=w1287) -> ("dup refnum"=w1284:refnum<file>, "error out"=w1285:errorcluster)  [unwired: 1 in]
        n338 = Close File(refnum=w1284, error in=w1285) -> (error out=w1273:errorcluster)  [unwired: 1 out]
      }
      frame "serial" {
        n339 = local read "Enable Termination\nChar (T)"() -> (w1337:bool)
        n340 = local read "Termination char\n(0xA = '\\n' = LF)\n(0xD = '\\r' = CR)"() -> (w1336:u8)
        n341 = Index Array(array=w1344, index=0 ("Index")) -> (element=w1343:string)
        n342 = local read "parity"() -> (w1327:u16)
        n343 = local read "Delay before read (ms)"() -> (w1338:u32)
        n344 = local read "byte count"() -> (w1335:u32)
        n345 = local read "Timeout (ms)"() -> (w1334:u32)
        n346 = local read "VISA resource name"() -> (w1331:refnum<visa-resource-name>)
        n347 = local read "baud rate"() -> (w1330:u32)
        n348 = local read "Serial End Mode for Reads"() -> (w1329:u16)
        n349 = local read "data bits"() -> (w1328:u16)
        n350 = local read "stop bits"() -> (w1333:u16)
        n351 = local read "flow control"() -> (w1332:u16)
        n352 = call "Serial write and read v0.5.vi"("Delay before read (ms)"=w1338, "Termination char\n(0xA = '\\n' = LF)\n(0xD = '\\r' = CR)"=w1336, "Enable Termination\nChar (T)"=w1337, "parity"=w1327, "stop bits"=w1333, "string to write"=w1343, "flow control"=w1332, "byte count"=w1335, "Serial Settings:Serial End Mode for Reads"=w1329, "Timeout (ms)"=w1334, "error in (no error)"=w1349, "VISA resource name"=w1331, "baud rate"=w1330, "data bits"=w1328) -> ("Serial port output"=w1339:string, "error out"=w1348:errorcluster)
        n353 = Build Array (concatenate)(w1339, w1340) -> (w1341:string[])
      }
      frame "pump" {
        # "Time array for absolute plunger position"
        # "Absolute plunger position"
        # "Remove \"_\""
        # "Check if hard stop is pressed."
        # "Check if halt is pressed."
        # "Check if pump is idle. Else halt."
        n354 = local read "Hard stop pump"() -> (w1377:bool)
        n355 = local read "Halt pump"() -> (w1380:bool)
        n356 = local read "Enable Termination\nChar (T)"() -> (w1394:bool)
        n357 = local read "Termination char\n(0xA = '\\n' = LF)\n(0xD = '\\r' = CR)"() -> (w1393:u8)
        n358 = Index Array(array=w1398, index=0 ("Index")) -> (element=w1375:string)
        n359 = case shown="\"Initialization\"" w1373 {
          tunnel: w1375 -> [w1429 _ w1431 w1432 w1433 w1434 _ _ w1437 w1438 _]
          tunnel: [w1429 "/1H" w1431 w1432 w1433 w1434 "/1H" "/1H" w1437 w1438 "/1H"] -> w1374
          frame "No error", Default {
          }
          frame "Initialization" {
          }
          frame "Invalid command" {
          }
          frame "Invalid operand" {
          }
          frame "Device not initialized" {
          }
          frame "Internal failure" {
          }
          frame "Plunger overload" {
          }
          frame "Valve overload" {
          }
          frame "Plunger move not allowed" {
          }
          frame "A/D converter failure" {
          }
          frame "Command overflow" {
          }
        }
        n360 = case shown="True" w1380 {
          tunnel: [w1443 "/1H"] -> w1379
          tunnel: w1374 -> [w1443 _]
          frame False {
          }
          frame True {
            n361 = local write "Halt pump"(FALSE) -> ()
          }
        }
        n362 = case shown="True" w1377 {
          tunnel: [w1440 "/1T"] -> w1378
          tunnel: w1379 -> [w1440 _]
          frame False {
          }
          frame True {
            n363 = local write "Hard stop pump"(FALSE) -> ()
          }
        }
        n364 = local read "Serial End Mode for Reads"() -> (w1386:u16)
        n365 = local read "flow control"() -> (w1389:u16)
        n366 = local read "stop bits"() -> (w1390:u16)
        n367 = local read "parity"() -> (w1384:u16)
        n368 = local read "Delay before read (ms)"() -> (w1395:u32)
        n369 = local read "byte count"() -> (w1392:u32)
        n370 = local read "Timeout (ms)"() -> (w1391:u32)
        n371 = local read "VISA resource name"() -> (w1388:refnum<visa-resource-name>)
        n372 = local read "baud rate"() -> (w1387:u32)
        n373 = local read "data bits"() -> (w1385:u16)
        n374 = String Subset(string=w1369, offset (0)=1) -> (substring=w1367:string)  [unwired: 1 in]
        n375 = call "SPM Pump v0.5.vi"("Termination char\n(0xA = '\\n' = LF)\n(0xD = '\\r' = CR)"=w1393, "Enable Termination\nChar (T)"=w1394, "Timeout (ms)"=w1391, "Serial Settings:Serial End Mode for Reads"=w1386, "byte count"=w1392, "Delay before read (ms)"=w1395, "Time <input>"=w1372, "error in (no error)"=w1403, "Serial port input"=w1378, "VISA resource name"=w1388, "parity"=w1384, "baud rate"=w1387, "stop bits"=w1390, "data bits"=w1385, "flow control"=w1389, "Time units <input>"=w1367) -> ("Input Command"=w1366:string, "Pump status"=w1362:string, "Valve position"=w1364:i32, "Absolute plunger position"=w1376:i32, "Serial port output"=w1371:string, "error out"=w1402:errorcluster)  [unwired: 2 in, 4 out]
        n376 = case shown="\"Q\", Default" w1366 {
          tunnel: [w1414 w1421 w1424] -> w1383
          tunnel: w1382 -> [w1414 w1420 w1424]
          tunnel: w1376 -> [_ w1419 _]
          tunnel: w1363 -> [w1413 w1418 w1425]
          tunnel: [w1413 w1418 w1427] -> w1365
          tunnel: w1364 -> [_ _ w1426]
          tunnel: w1361 -> [_ w1417 _]
          tunnel: w1360 -> [w1412 w1416 w1423]
          tunnel: [w1412 w1415 w1423] -> w1359
          frame "Q", Default {
          }
          frame "?" {
            n377 = Build Array (concatenate)(w1420, w1419) -> (w1421:i32[])
            n378 = Build Array (concatenate)(w1416, w1417) -> (w1415:i32[])
            n379 = call "4155C Split array.vi"("X data in"=w1415, "Y1 data in"=w1421) -> ("Array of clusters"=w1422:cluster{"Y data in":dbl[], "X data in":dbl[]}[])  [unwired: 5 in, 1 out]
            n380 = local write "Absolute plunger position vs time"(w1422) -> ()
          }
          frame "?6" {
            n381 = Build Array (concatenate)(w1425, w1426) -> (w1427:i32[])
            n382 = call "4155C Split array.vi"("Y1 data in"=w1427) -> ("Array of clusters"=w1428:cluster{"Y data in":dbl[], "X data in":dbl[]}[])  [unwired: 6 in, 1 out]
            n383 = local write "Valve position vs time"(w1428) -> ()
          }
        }
        n384 = Build Array (concatenate)(w1370, w1371) -> (w1396:string[])
      }
    }
    n385 = Build Array(w55, w106, w100) -> (w105:dbl[][])
    n386 = Build Array(w50, w56) -> (w64:i32[][])
    n387 = Concatenate Strings(w53, "Prefix (serial port output)", ".txt" ("Suffix")) -> (w82:string)
    n388 = Build Array(w57, "Id max /A" ("VAR2 Name"), "Id min /A" ("VAR2 Name")) -> (w111:string[])
    n389 = Build Array(w57, "Absolute plunger position" ("VAR2 Name")) -> (w67:string[])
    n390 = Array To Spreadsheet String(array=w83, 3:"" ("format string")) -> (spreadsheet string=w88:string)  [unwired: 1 in]
    n391 = Transpose 2D Array(2D array=w105) -> (transposed array=w104:dbl[][])
    n392 = Transpose 2D Array(2D array=w64) -> (transposed array=w54:i32[][])
    n393 = String To Path(string=w82) -> (path=w79:path)
    n394 = Concatenate Strings(w53, "Prefix (Idmax-Idmin)", "Suffix (Idmax-Idmin)") -> (w118:string)
    n395 = Array To Spreadsheet String(array=w67, 3:"" ("format string")) -> (spreadsheet string=w66:string)  [unwired: 1 in]
    n396 = Array To Spreadsheet String(array=w111, 3:"" ("format string")) -> (spreadsheet string=w110:string)  [unwired: 1 in]
    n397 = Array To Spreadsheet String(array=w104, 3:"%e" ("format string")) -> (spreadsheet string=w109:string)  [unwired: 1 in]
    n398 = Array To Spreadsheet String(array=w54, 3:"%e" ("format string")) -> (spreadsheet string=w63:string)  [unwired: 1 in]
    n399 = String To Path(string=w118) -> (path=w117:path)
    n400 = local write "Serial port data"(w88) -> ()
    n401 = Write to Text File(file (use dialog)=w79, text=w83, error in=w78) -> (refnum out=w84:refnum<file>, error out=w85:errorcluster)  [unwired: 1 in, 1 out]
    n402 = Build Array(w66, w63) -> (w69:string[])
    n403 = Build Array(w110, w109) -> (w108:string[])
    n404 = Close File(refnum=w84, error in=w85) -> (error out=w77:errorcluster)  [unwired: 1 out]
    n405 = Concatenate Strings(w53, "Prefix (plunger)", "Suffix (plunger)") -> (w61:string)
    n406 = String To Path(string=w61) -> (path=w58:path)
    n407 = Write to Text File(file (use dialog)=w117, text=w108, error in=w77) -> (refnum out=w119:refnum<file>, error out=w107:errorcluster)  [unwired: 1 in, 1 out]
    n408 = Write to Text File(file (use dialog)=w58, text=w69) -> (refnum out=w62:refnum<file>, error out=w71:errorcluster)  [unwired: 2 in, 1 out]
    n409 = Close File(refnum=w119, error in=w107) -> (error out=w102:errorcluster)  [unwired: 1 out]
    n410 = Close File(refnum=w62, error in=w71) -> ()  [unwired: 2 out]
  }
  "error out" <- w9
